vi "New Template - Test Plan Template (SubVI).vi"(8 "error in":errorcluster, 9 "Load path":path, 10 "File Name:":string, 11 "Test Type":T1 items=["Please Select", "Triaxial Shear", "Triaxial UU", "Shearbox", "Permeability", "Consolidation (Stepped Loading)/Swelling", "Saturation (Incremental)", "User Defined", "UCT", "Isotropic Consolidation", "Swelling Pressure"]) -> (0 "error out":errorcluster)   [LabVIEW 2019]
uses:
  Controls/Test Plan - Start Conditions Tab.ctl
  Controls/Test Plan - Stop Conditions Tab.ctl
  Controls/Test Plan - Log Conditions Tab.ctl
  Controls/Station - Test Type.ctl
  Controls/Test Plan Template - State.ctl
panel:
  in  "Save":bool
  in  "Tab con":T2(tab)
  in  "Start Enable":bool
  out "Start Tab":T3=enum."User Defined"
  in  "Cons Start VS":dbl caption="N"
  in  "Cons Start Delay":timestamp format="%<%H:%M:%S>T"
  in  "Cons Start .Delay":bool
  in  "Sat Start BP":bool
  in  "Sat BP":dbl caption="kPa"
  in  "Sat CP":dbl caption="kPa"
  in  "Iso BP":dbl caption="kPa"
  in  "Start Load":string[][](table) caption="Use the following table for consolidation pressure:"
  in  "Start load":dbl format="%#_13g"
  in  "Start Delay":u32
  in  "Sub Start":enum32{"1", "2"}(radio)
  in  "TS Drain":enum32{"1", "2"}(radio)
  in  "TS Engage":bool
  in  "TS Load Change":dbl caption="N"
  in  "TS Engage Speed":dbl caption="mm/min"
  in  "TS Shear Speed":dbl caption="mm/min"
  in  "TUU Start Delay":timestamp format="%<%H:%M:%S>T"
  in  "TUU Start .Delay":bool
  in  "TUU Confining Pressure":dbl caption="kPa"
  in  "TUU Engage":bool
  in  "TUU Load Change":dbl caption="N"
  in  "TUU Engage Speed":dbl caption="mm/min"
  in  "TUU Shear Speed":dbl caption="mm/min"
  in  "UCT Engage":bool
  in  "UCT Load Change":dbl caption="N"
  in  "UCT Engage Speed":dbl caption="mm/min"
  in  "UCT Shear Speed":dbl caption="mm/min"
  in  "SB Start Delay":timestamp format="%<%H:%M:%S>T"
  in  "SB Start .Delay":bool
  in  "SB Vertical Load":dbl caption="N"
  in  "SB Engage":bool
  in  "SB Load Change":dbl caption="N"
  in  "SB Engage Speed":dbl caption="mm/min"
  in  "SB Shear Speed":dbl caption="mm/min"
  in  "Perm DP":dbl caption="kPa"
  out "Log Tab":T4=enum."User Defined"
  in  "Cons Log Select":enum32{"1", "2"}(radio)
  out "ConsTable":enum32{"None", "Time", "Disp"}(tab)
  in  "Cons LogTime":string[][](table)
  in  "Cons LogDisp":string[][](table)
  in  "Cons Log Delay":timestamp format="%<%H:%M:%S>T"
  in  "Sat Log Delay":timestamp format="%<%H:%M:%S>T"
  out "SatTable":enum32{"None", "Time", "Disp"}(tab)
  in  "Sat LogTime":string[][](table)
  in  "Sat LogDisp":string[][](table)
  in  "Sat Log Select":enum32{"1", "2"}(radio)
  in  "Iso Log Select":enum32{"1", "2"}(radio)
  out "IsoTable":enum32{"None", "Time", "Disp"}(tab)
  in  "Iso LogTime":string[][](table)
  in  "Iso LogDisp":string[][](table)
  in  "Iso Log Delay":timestamp format="%<%H:%M:%S>T"
  in  "LOG delay":u32
  out "LOG Table":enum32{"None", "Time", "Disp"}(tab)
  in  "LOG Time":string[][](table)
  in  "LOG Disp":string[][](table)
  in  "Sub Log":enum32{"1", "2", "3"}(radio)
  in  "Log VL":u16(ring) caption="Vertical Load(Kpa)" items=["Please select"]
  in  "SET":bool
  in  "TS LogAxial":sgl
  in  "TS Log Delay":timestamp format="%<%H:%M:%S>T"
  out "TSTable":enum32{"None", "Time", "Disp"}(tab)
  in  "TS LogTime":string[][](table)
  in  "TS LogDisp":string[][](table)
  in  "TS Log Select":enum32{"1", "3", "2"}(radio)
  in  "TUU LogAxial":sgl
  in  "TUU Log Delay":timestamp format="%<%H:%M:%S>T"
  out "TUUTable":enum32{"None", "Time", "Disp"}(tab)
  in  "TUU LogTime":string[][](table)
  in  "TUU LogDisp":string[][](table)
  in  "TUU Log Select":enum32{"1", "3", "2"}(radio)
  in  "UCT LogAxial":sgl
  in  "UCT Log Delay":timestamp format="%<%H:%M:%S>T"
  out "UCTTable":enum32{"None", "Time", "Disp"}(tab)
  in  "UCT LogTime":string[][](table)
  in  "UCT LogDisp":string[][](table)
  in  "UCT Log Select":enum32{"1", "3", "2"}(radio)
  in  "SB Log Delay":timestamp format="%<%H:%M:%S>T"
  out "SBTable":enum32{"None", "Time", "Disp"}(tab)
  in  "SB LogTime":string[][](table)
  in  "SB LogDisp":string[][](table)
  in  "SB Log Select":enum32{"1", "2"}(radio)
  in  "Perm Log Delay":timestamp format="%<%H:%M:%S>T"
  in  "Perm Log Select":enum32{"1"}(radio)
  in  "SP Log Delay":timestamp format="%<%H:%M:%S>T"
  in  "SP Log Select":enum32{"1"}(radio)
  in  "Stop Enable":bool
  out "Stop Tab":T5=enum."User Defined"
  in  "Cons Stop Swell":bool caption="When swelling is detected by the amount given"
  in  "Cons Stop Time":timestamp format="%<%H:%M:%S>T"
  in  "Cons Stop Time2":string="00:00:00"
  in  "Cons Stop Select":enum32{"1", "2"}(radio)
  in  "Cons Stop Disp":dbl caption="mm"
  in  "Cons Stop Disp 2":dbl caption="mm"
  in  "Sat Stop Time3":string="00:00:00"
  in  "Sat Stop VC":dbl caption="cm3"
  in  "Sat Stop PP":dbl caption="kPa"
  in  "Sat Stop Select":enum32{"1", "2", "3"}(radio)
  in  "Sat Stop Time2":timestamp format="%<%H:%M:%S>T"
  in  "Sat Stop Time":timestamp format="%<%H:%M:%S>T"
  in  "Sat Stop B":dbl caption="%" format="%.2f"
  in  "Sat Stop .B":bool
  in  "Iso Stop Time":string="00:00:00"
  in  "Iso Stop Select":enum32{"1", "2"}(radio)
  in  "Iso Stop Time2":timestamp format="%<%H:%M:%S>T"
  in  "Iso Stop PP":dbl caption="%"
  in  "Iso Stop VC":dbl caption="cm3"
  in  "Iso Stop .PP":bool
  in  "Return":bool
  in  "Stop Time":timestamp=timestamp(57600 s since 1904-01-01) format="%<%H:%M:%S>T"
  in  "Stop Duration":u32
  in  "stop load":dbl format="%#_13g"
  in  "Sub Stop":enum32{"1", "2"}(radio)
  in  "TS Reset Value":dbl caption="%"
  in  "TS Axial Value":dbl caption="%"
  in  "TS MaxDev":bool
  in  "TS MaxDev Value":dbl caption="%"
  in  "TS Reset":bool
  in  "TS Return":bool
  in  "TUU Reset Value":dbl caption="%"
  in  "TUU Axial Value":dbl caption="%"
  in  "TUU MaxDev":bool
  in  "TUU MaxDev Value":dbl caption="%"
  in  "TUU Reset":bool
  in  "TUU Return":bool
  in  "UCT Reset Value":dbl caption="%"
  in  "UCT Axial Value":dbl caption="%"
  in  "UCT MaxDev":bool
  in  "UCT MaxDev Value":dbl caption="%"
  in  "UCT Reset":bool
  in  "UCT Return":bool
  in  "SB Reset Value":dbl caption="%"
  in  "SB Shear Value":dbl caption="%"
  in  "SB MaxShear":bool
  in  "SB MaxShear Value":dbl caption="%"
  in  "SB Reset":bool
  in  "SB Return":bool
  in  "Perm Ratio More":dbl caption="%"
  in  "Perm Ratio Time":string="00:00:00"
  in  "Perm Stop Time":string="00:00:00"
  in  "Perm Reset Value":dbl caption="%"
  in  "Perm Ratio Less":dbl caption="%"
  in  "Perm MaxTime":bool
  in  "Perm Reset":bool
  in  "Perm Ratio":bool
  in  "SP Stop Time":string="00:00:00"
  in  "SP Stop Max Time":string="00:00:00"
  in  "SP Stop Stress":dbl caption="%"
  in  "SP Stop .MaxTime":bool
  in  "SP Stop .Time":bool
  # "Vertical Load will be :"
  # "Wait until the following delay expires"
  # "Cell Pressure will be :"
  # "Back Pressure will be :"
  # "Hold Back Pressure at :"
  # "Shear speed will be:"
  # "Engage Speed :"
  # "Until the load changes by"
  # "Wait until the following delay expires"
  # "Confining Pressure will be:"
  # "Shear speed will be:"
  # "Engage Speed :"
  # "Until the load changes by"
  # "Shear speed will be:"
  # "Engage Speed :"
  # "Until the load changes by"
  # "Wait until the following delay expires"
  # "Vertical Load will be:"
  # "Shear speed will be:"
  # "Engage Speed :"
  # "Until the load changes by"
  # "Drain Pressure will be:"
  # "Data will be logged as soon as the test is started"
  # "B value is above this level"
  # "When the Pore Pressure Dissipation exceeds the\npercentage entered here"
  # "When the Axial Strain extends beyond the\npercentage entered here"
  # "When the Maximum Deviator Stress falls by the\npercentage entered here"
  # "Return the load frame to home position"
  # "Reset Cell And Back Pressure Control to amount\nentered here"
  # "When the Axial Strain extends beyond the\npercentage entered here"
  # "When the Maximum Deviator Stress falls by the\npercentage entered here"
  # "Return the load frame to home position"
  # "Reset Cell Pressure Control to amount\nentered here"
  # "When the Axial Strain extends beyond the\npercentage entered here"
  # "When the Maximum Deviator Stress falls by the\npercentage entered here"
  # "Return the load frame to home position"
  # "When the Shear Strain extends beyond the\npercentage entered here"
  # "When the Maximum Shear Stress falls by the\npercentage entered here"
  # "Return the Horizontal piston to home position"
  # "Reset Vertical Load to amount\nentered here"
  # "<= Ratio <="
  # "When the top and bottom volume change is steady\n(constant flow) over the period of time entered here"
  # "When the maximum time entered here is exceeded"
  # "Reset Drain Pressure, Back Pressure and\nCell Pressure to amount entered here"
  # "Stop when the Specimen Stress Changes by less  than \nthis amount during the following interval : (kPa/time)"
  # "When the maximum time entered here is exceeded"
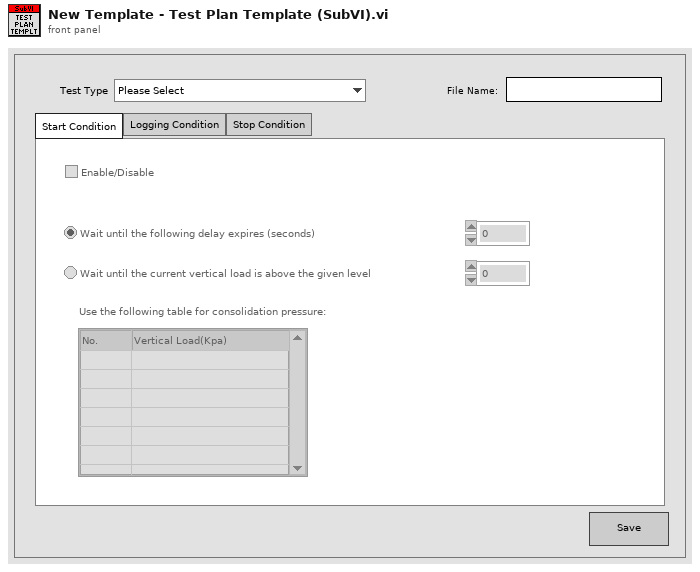
[diagram p1: front panel]
types:
  T1 = typedef "Station - Test Type.ctl" = u16
  T2 = enum32{"Start Condition", "Logging Condition", "Stop Condition"}
  T3 = typedef "Test Plan - Start Conditions Tab.ctl" = enum32{"Consolidation", "Saturation", "Iso Consolidation", "User Defined", "Others", "TS", "TUU", "UCT", "Shearbox", "Permiability", "SP"}
  T4 = typedef "Test Plan - Log Conditions Tab.ctl" = enum32{"Consolidation", "Saturation", "Iso Consolidation", "User Defined", "Others", "TS", "TUU", "UCT", "Shearbox", "Permiability", "SP"}
  T5 = typedef "Test Plan - Stop Conditions Tab.ctl" = enum32{"Consolidation", "Saturation", "Iso Consolidation", "User Defined", "Others", "TS", "TUU", "UCT", "Shearbox", "Permiability", "SP"}
  T6 = typedef "Test Plan Template - State.ctl" = enum16{"Init", "Idle", "Load VL", "Load Start", "Load Log", "Load Stop", "Load Device", "Save", "Close"}
  T7 = enum8{"Enabled", "Disabled", "Disabled and Grayed Out"}
  T8 = cluster{"TestPlan Section":string, "Key Value":string[]}[]
  T9 = cluster{"TestPlan Section":string, "Key Value":string[]}
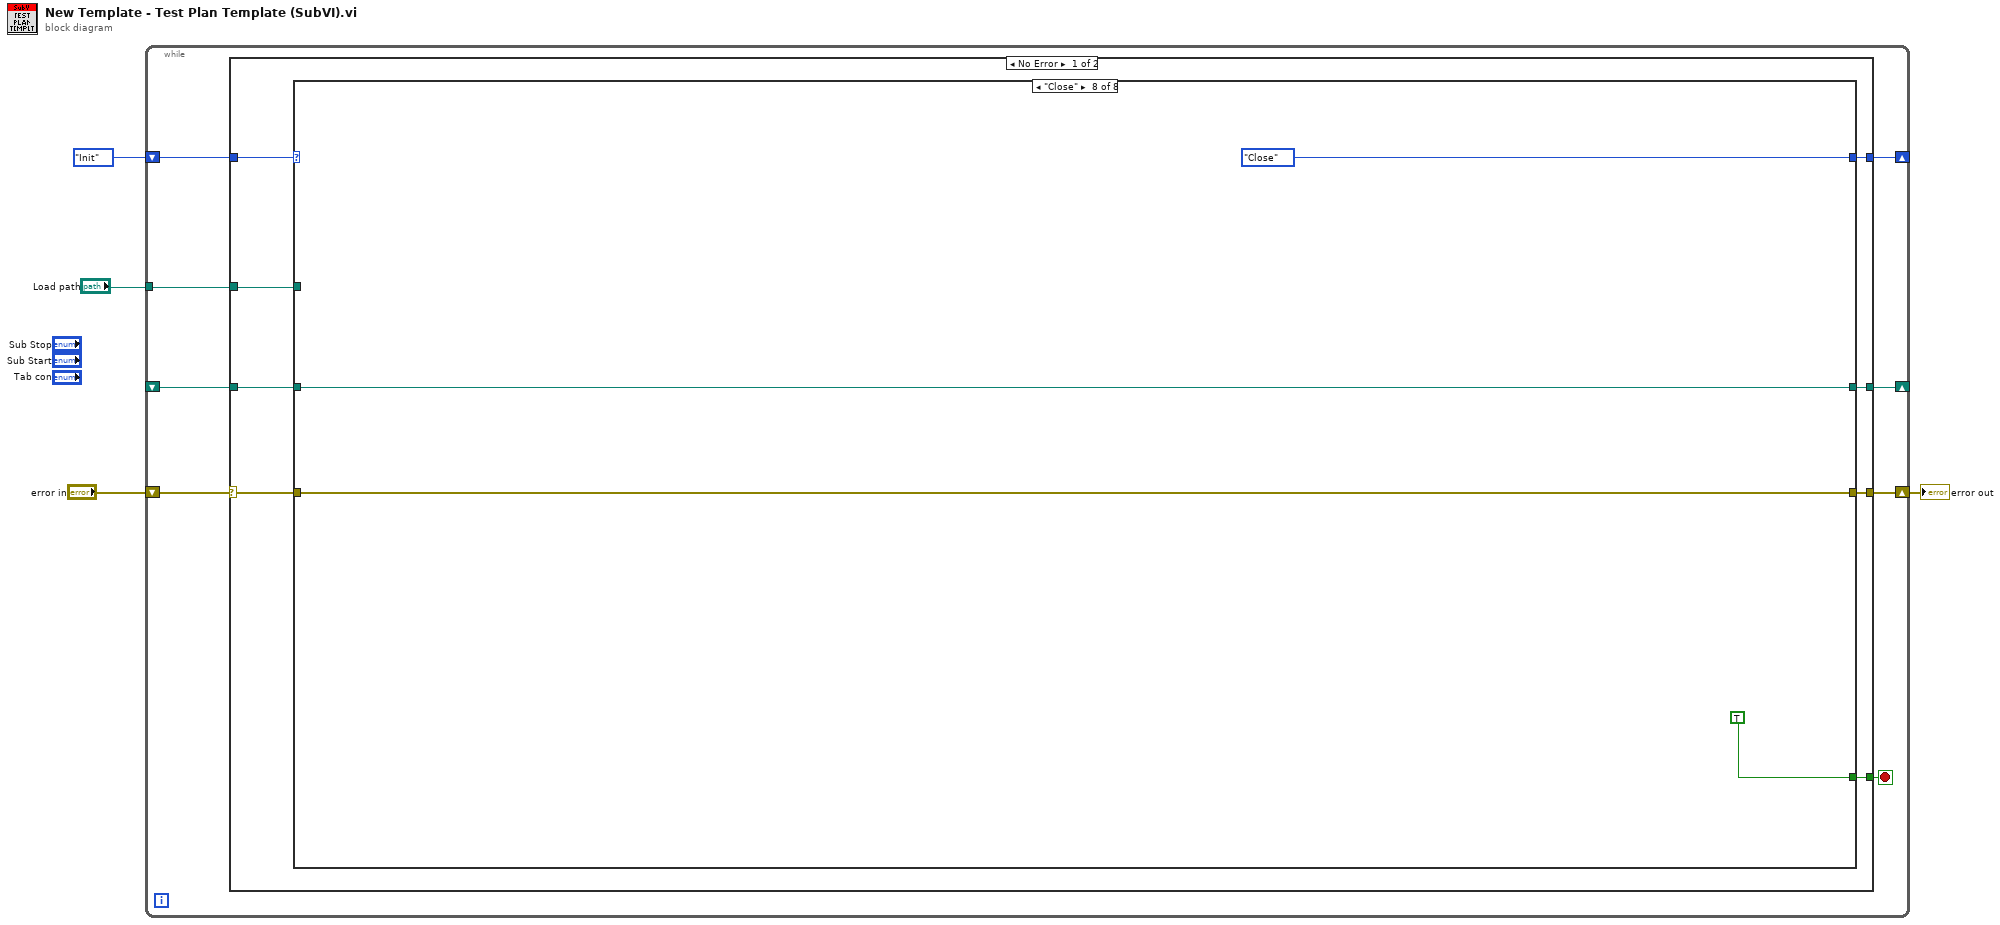
[diagram p0: block diagram]
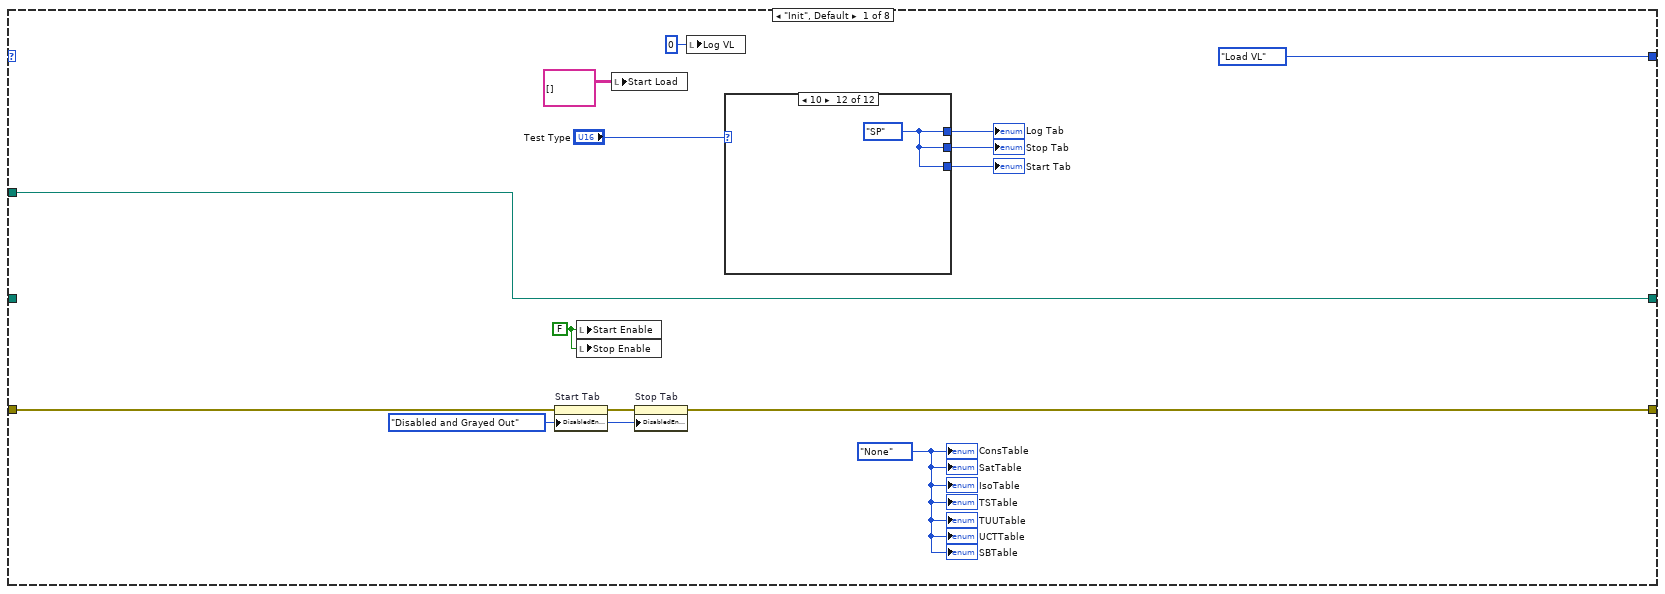
[diagram p2: hidden frame]
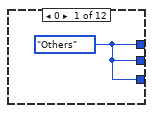
[diagram p3: hidden frame]
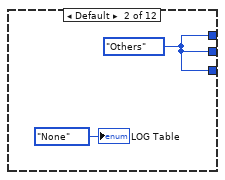
[diagram p4: hidden frame]
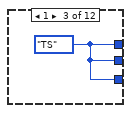
[diagram p5: hidden frame]
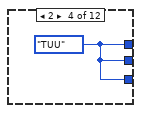
[diagram p6: hidden frame]
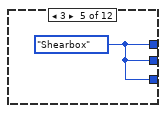
[diagram p7: hidden frame]
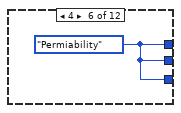
[diagram p8: hidden frame]
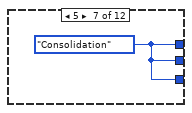
[diagram p9: hidden frame]
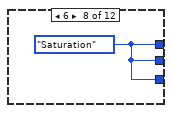
[diagram p10: hidden frame]
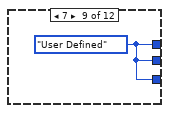
[diagram p11: hidden frame]
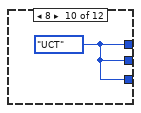
[diagram p12: hidden frame]
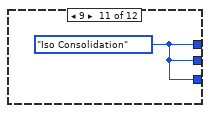
[diagram p13: hidden frame]
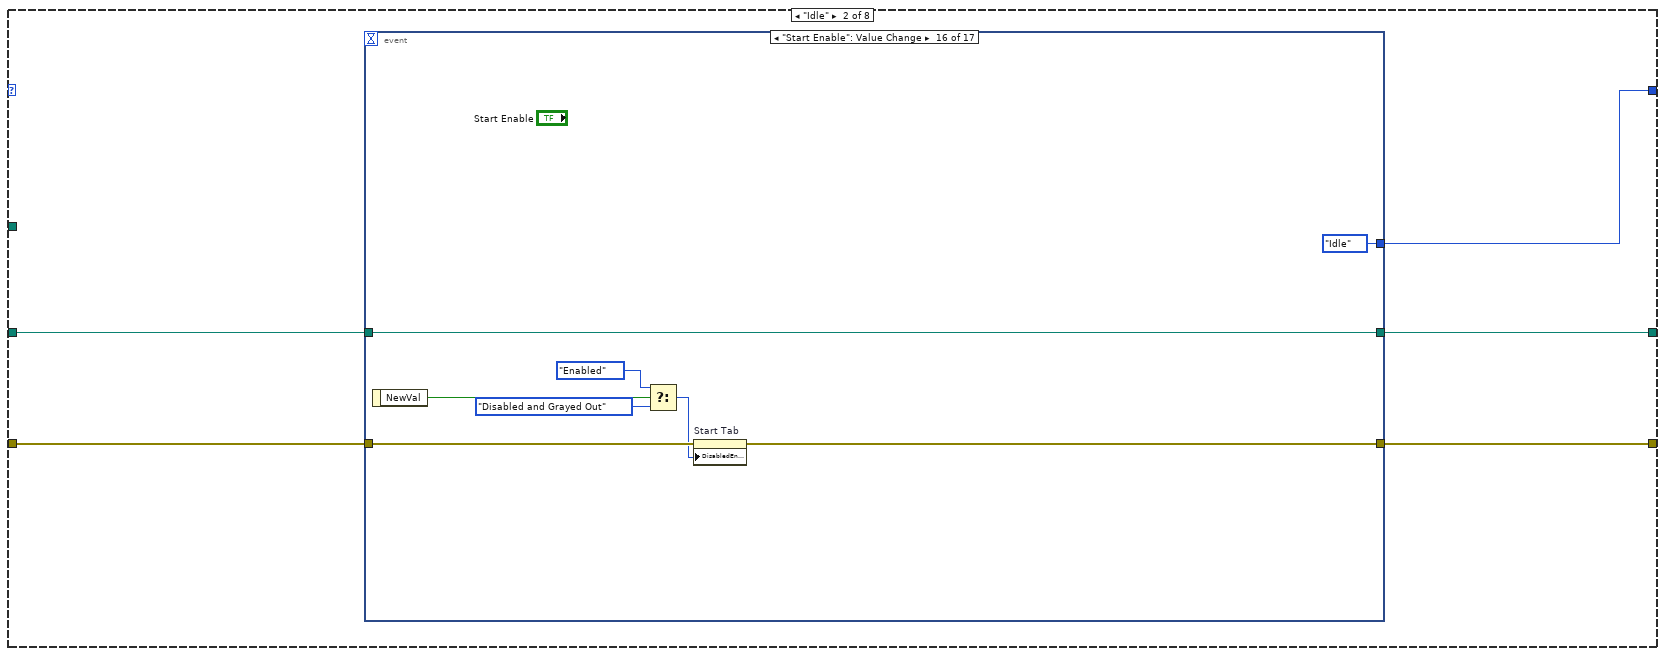
[diagram p14: hidden frame]
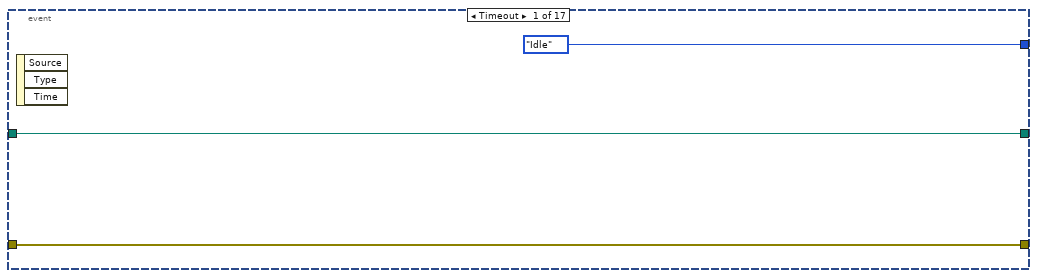
[diagram p15: hidden frame]
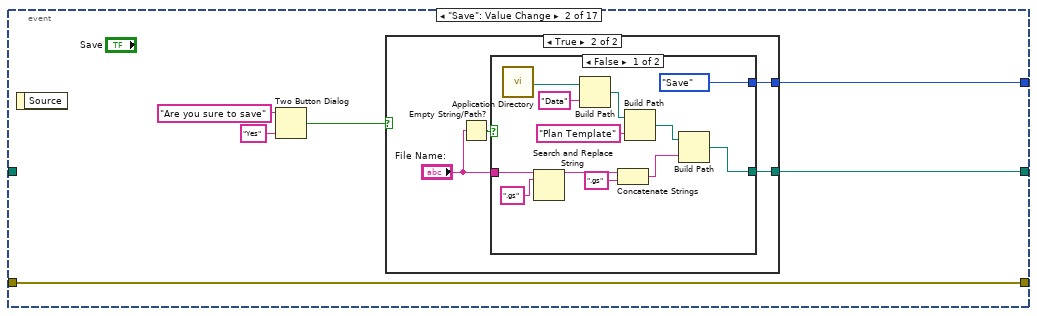
[diagram p16: hidden frame]
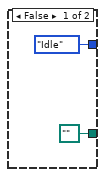
[diagram p17: hidden frame]
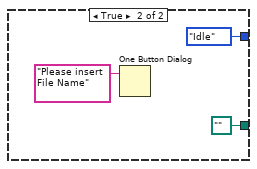
[diagram p18: hidden frame]
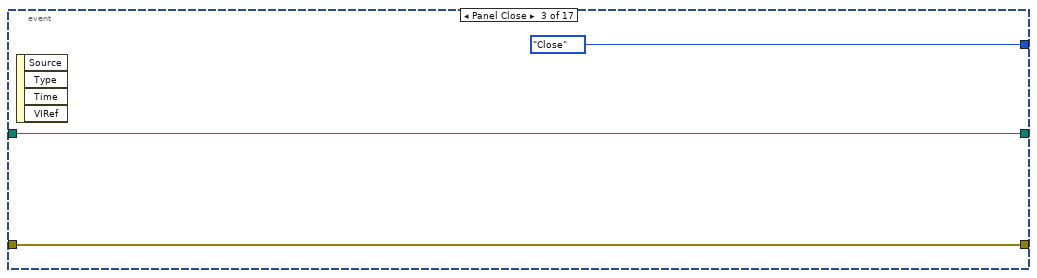
[diagram p19: hidden frame]
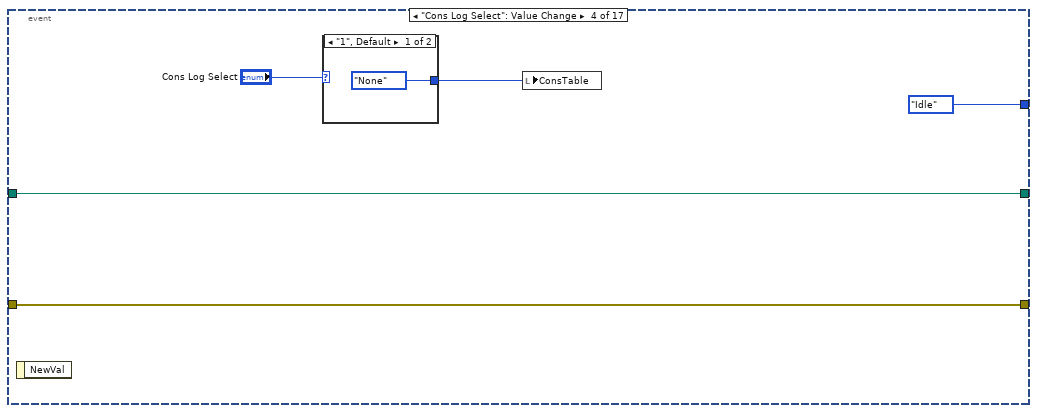
[diagram p20: hidden frame]
diagram:
  n1 = while {
    shift-right: [w12] -> w4
    shift-left: "error in" -> [w11]
    shift-right: [w9] -> _
    shift-left: Test_Plan_Template_-_State."Init" -> [w10]
    shift-right: [w8] -> _
    shift-left: _ -> [w7]
    tunnel: "Load path" -> [w5]
    stop <- w6 stop-if-true
    n2 = case shown="No Error" w11 {
      selector: w11 -> [w19 w1656]
      tunnel: [w20 w1655] -> w12
      tunnel: w10 -> [w18 _]
      tunnel: [w17 Test_Plan_Template_-_State."Idle" ("Enum")] -> w9
      tunnel: [w16 w1652] -> w8
      tunnel: w7 -> [w15 w1652]
      tunnel: [w14 _] -> w6
      tunnel: w5 -> [w13 _]
      frame No Error {
        n3 = case shown="\"Close\"" w18 {
          tunnel: [w24 w52 w264 w291 w471 w789 w1121 w1651] -> w20
          tunnel: w19 -> [w23 w51 w269 w296 w476 w794 w1126 w1651]
          tunnel: [Test_Plan_Template_-_State."Load VL" w50 Test_Plan_Template_-_State."Load Start" ("Enum") Test_Plan_Template_-_State."Load Log" ("Enum") Test_Plan_Template_-_State."Load Stop" ("Enum") Test_Plan_Template_-_State."Idle" ("Enum") w1120 Test_Plan_Template_-_State."Close" ("Enum")] -> w17
          tunnel: [w30 w49 w266 w293 w473 w791 w1123 w1650] -> w16
          tunnel: w15 -> [_ w48 w265 w292 w472 w790 w1123 w1650]
          tunnel: [_ _ _ _ _ _ _ TRUE] -> w14
          tunnel: w13 -> [w30 _ w268 w295 w475 w793 _ _]
          frame "Init", Default {
            w22 = T7."Disabled and Grayed Out" ("Disabled")
            w26 = FALSE ("Start Enable")
            w21 = enum32{"None", "Time", "Disp"}."None" ("CustomTable")
            n4 = property on="Start Tab" class="TabCtl (strict)"(error in=w23, "DisabledEnum"=w22) -> (error out=w25:errorcluster)  [unwired: 1 in, 1 out]
            n5 = local write "Start Enable"(w26) -> ()
            n6 = local write "Stop Enable"(w26) -> ()
            n7 = local write "Start Load"(string[][] [] ("Start 1DLoad")) -> ()
            n8 = property on="Stop Tab" class="TabCtl (strict)"(error in=w25, "DisabledEnum"=w22) -> (error out=w24:errorcluster)  [unwired: 1 in, 1 out]
            n9 = local write "Log VL"(0) -> ()
            n10 = case shown="10" "Test Type" {
              tunnel: [w35 w36 w38 w39 w40 w41 w42 w43 w44 w45 w46 w47] -> w29
              tunnel: [w35 w36 w38 w39 w40 w41 w42 w43 w44 w45 w46 w47] -> w28
              tunnel: [w35 w36 w38 w39 w40 w41 w42 w43 w44 w45 w46 w47] -> w27
              frame 0 {
                w35 = Test_Plan_-_Log_Conditions_Tab."Others" ("Log Tab")
              }
              frame Default {
                w36 = Test_Plan_-_Log_Conditions_Tab."Others" ("Log Tab")
                "LOG Table" <- enum32{"None", "Time", "Disp"}."None" ("1DTable")
              }
              frame 1 {
                w38 = Test_Plan_-_Log_Conditions_Tab."TS" ("Log Tab")
              }
              frame 2 {
                w39 = Test_Plan_-_Log_Conditions_Tab."TUU" ("Log Tab")
              }
              frame 3 {
                w40 = Test_Plan_-_Log_Conditions_Tab."Shearbox" ("Log Tab")
              }
              frame 4 {
                w41 = Test_Plan_-_Log_Conditions_Tab."Permiability" ("Log Tab")
              }
              frame 5 {
                w42 = Test_Plan_-_Log_Conditions_Tab."Consolidation" ("Log Tab")
              }
              frame 6 {
                w43 = Test_Plan_-_Log_Conditions_Tab."Saturation" ("Log Tab")
              }
              frame 7 {
                w44 = Test_Plan_-_Log_Conditions_Tab."User Defined" ("Log Tab")
              }
              frame 8 {
                w45 = Test_Plan_-_Log_Conditions_Tab."UCT" ("Log Tab")
              }
              frame 9 {
                w46 = Test_Plan_-_Log_Conditions_Tab."Iso Consolidation" ("Log Tab")
              }
              frame 10 {
                w47 = Test_Plan_-_Log_Conditions_Tab."SP" ("Log Tab")
              }
            }
            "Log Tab" <- w29
            "Stop Tab" <- w28
            "Start Tab" <- w27
            "ConsTable" <- w21
            "SatTable" <- w21
            "IsoTable" <- w21
            "TSTable" <- w21
            "TUUTable" <- w21
            "UCTTable" <- w21
            "SBTable" <- w21
          }
          frame "Idle" {
            n11 = event shown="[15] \"Start Enable\": Value Change" {
              selector: _ -> [_ _ _ _ _ _ _ _ _ _ _ _ _ _ _ _ _]
              dyn-events: _ -> [_ _ _ _ _ _ _ _ _ _ _ _ _ _ _ _ _]
              timeout: _ -> [_ _ _ _ _ _ _ _ _ _ _ _ _ _ _ _ _]
              tunnel: [w55 w60 w85 w88 w95 w102 w109 w116 w123 w128 w131 w136 w141 w215 w246 w253 w259] -> w52
              tunnel: w51 -> [w55 w60 w85 w88 w95 w102 w109 w116 w123 w128 w131 w136 w152 w237 w246 w252 w258]
              tunnel: [Test_Plan_Template_-_State."Idle" w61 Test_Plan_Template_-_State."Close" ("Enum") Test_Plan_Template_-_State."Idle" ("Enum") Test_Plan_Template_-_State."Idle" ("Enum") Test_Plan_Template_-_State."Idle" ("Enum") Test_Plan_Template_-_State."Idle" ("Enum") Test_Plan_Template_-_State."Idle" ("Enum") Test_Plan_Template_-_State."Idle" ("Enum") Test_Plan_Template_-_State."Idle" ("Enum") Test_Plan_Template_-_State."Idle" ("Enum") Test_Plan_Template_-_State."Idle" ("Enum") Test_Plan_Template_-_State."Idle" ("Enum") Test_Plan_Template_-_State."Idle" ("Enum") Test_Plan_Template_-_State."Idle" ("Enum") Test_Plan_Template_-_State."Idle" ("Enum") Test_Plan_Template_-_State."Idle" ("Enum")] -> w50
              tunnel: [w53 w59 w84 w90 w97 w104 w111 w118 w125 w130 w133 w138 w151 w216 w247 w255 w263] -> w49
              tunnel: w48 -> [w53 _ w84 w90 w97 w104 w111 w118 w125 w130 w133 w138 w151 w216 w247 w255 w263]
              event Timeout {
                n12 = event-data() -> ()  [unwired: 1 in, 3 out]
              }
              event "Save": Value Change {
                n13 = event-data() -> ()  [unwired: 1 in, 1 out]
                n14 = Two Button Dialog(message="Are you sure to save", 2:"Yes" ("T button name (\"OK\")")) -> (T button?=w58:bool)  [unwired: 1 in]
                n15 = case shown="True" w58 {
                  tunnel: [Test_Plan_Template_-_State."Idle" ("Enum") w67] -> w61
                  tunnel: [path "" ("appended path") w64] -> w59
                  frame False {
                  }
                  frame True {
                    n16 = Empty String/Path?(string/path="File Name:") -> (empty?=w65:bool)
                    n17 = case shown="False" w65 {
                      tunnel: [Test_Plan_Template_-_State."Save" ("Enum") Test_Plan_Template_-_State."Idle" ("Enum")] -> w67
                      tunnel: "File Name:" -> [w72 _]
                      tunnel: [w74 path "" ("appended path")] -> w64
                      frame False {
                        n18 = call <vilib>:"Application Directory.vi"() -> ("Application Directory"=w70:path)
                        n19 = Search and Replace String(input string=w72, search string=".gs") -> (result string=w73:string)  [unwired: 6 in, 3 out]
                        n20 = Build Path(base path=w70, name or relative path="Data") -> (appended path=w68:path)
                        n21 = Concatenate Strings(w73, ".gs" ("string")) -> (w78:string)
                        n22 = Build Path(base path=w68, name or relative path="Plan Template") -> (appended path=w77:path)
                        n23 = Build Path(base path=w77, name or relative path=w78) -> (appended path=w74:path)
                      }
                      frame True {
                        n24 = One Button Dialog(message="Please insert File Name") -> ()  [unwired: 1 in, 1 out]
                      }
                    }
                  }
                }
              }
              event Panel Close {
                n25 = event-data() -> ()  [unwired: 1 in, 4 out]
              }
              event "Cons Log Select": Value Change {
                n26 = event-data() -> ()  [unwired: 1 in, 1 out]
                n27 = case shown="\"1\", Default" "Cons Log Select" {
                  tunnel: [enum32{"None", "Time", "Disp"}."None" ("ConsTable") enum32{"None", "Time", "Disp"}."Time" ("ConsTable")] -> w86
                  frame "1", Default {
                  }
                  frame "2" {
                  }
                }
                n28 = local write "ConsTable"(w86) -> ()
              }
              event "Sat Log Select": Value Change {
                n29 = event-data() -> ()  [unwired: 1 in, 1 out]
                n30 = case shown="\"2\"" "Sat Log Select" {
                  tunnel: [enum32{"None", "Time", "Disp"}."None" ("ConsTable") enum32{"None", "Time", "Disp"}."Time" ("ConsTable")] -> w93
                  frame "1", Default {
                  }
                  frame "2" {
                  }
                }
                n31 = local write "SatTable"(w93) -> ()
              }
              event "Iso Log Select": Value Change {
                n32 = event-data() -> ()  [unwired: 1 in, 1 out]
                n33 = case shown="\"2\"" "Iso Log Select" {
                  tunnel: [enum32{"None", "Time", "Disp"}."None" ("ConsTable") enum32{"None", "Time", "Disp"}."Time" ("ConsTable")] -> w100
                  frame "1", Default {
                  }
                  frame "2" {
                  }
                }
                n34 = local write "IsoTable"(w100) -> ()
              }
              event "TS Log Select": Value Change {
                n35 = event-data() -> ()  [unwired: 1 in, 6 out]
                n36 = case shown="\"3\"" "TS Log Select" {
                  tunnel: [enum32{"None", "Time", "Disp"}."None" ("ConsTable") enum32{"None", "Time", "Disp"}."Disp" ("ConsTable")] -> w107
                  frame "1", Default {
                  }
                  frame "3" {
                  }
                }
                n37 = local write "TSTable"(w107) -> ()
              }
              event "TUU Log Select": Value Change {
                n38 = event-data() -> ()  [unwired: 1 in, 6 out]
                n39 = case shown="\"3\"" "TUU Log Select" {
                  tunnel: [enum32{"None", "Time", "Disp"}."None" ("ConsTable") enum32{"None", "Time", "Disp"}."Disp" ("ConsTable")] -> w114
                  frame "1", Default {
                  }
                  frame "3" {
                  }
                }
                n40 = local write "TUUTable"(w114) -> ()
              }
              event "SB Log Select": Value Change {
                n41 = event-data() -> ()  [unwired: 1 in, 6 out]
                n42 = case shown="\"2\"" "SB Log Select" {
                  tunnel: [enum32{"None", "Time", "Disp"}."None" ("ConsTable") enum32{"None", "Time", "Disp"}."Disp" ("ConsTable")] -> w122
                  frame "1", Default {
                  }
                  frame "2" {
                  }
                }
                n43 = local write "SBTable"(w122) -> ()
              }
              event "Perm Log Select": Value Change {
                n44 = event-data() -> ()  [unwired: 1 in, 6 out]
              }
              event "SP Log Select": Value Change {
                n45 = event-data() -> ()  [unwired: 1 in, 6 out]
              }
              event "UCT Log Select": Value Change {
                n46 = event-data() -> ()  [unwired: 1 in, 6 out]
                n47 = case shown="\"3\"" "UCT Log Select" {
                  tunnel: [enum32{"None", "Time", "Disp"}."None" ("ConsTable") enum32{"None", "Time", "Disp"}."Disp" ("ConsTable")] -> w134
                  frame "1", Default {
                  }
                  frame "3" {
                  }
                }
                n48 = local write "UCTTable"(w134) -> ()
              }
              event "Log VL": Value Change {
                n49 = event-data() -> ()  [unwired: 1 in, 1 out]
                n50 = call "TestPlan - Config File.vi"("Action"=enum16{"Write", "Read", "Read All", "Remove"}."Read", "file path"=w151, "error in (no error)"=w152, "TestPlan Section"="Log VL" ("TestPlan Name")) -> ("error out"=w149:errorcluster, "key names"=w146:string[], "Value Out"=w145:T8)  [unwired: 5 in]
                n51 = property on="Log VL" class="Ring (strict)"(error in=w149) -> (error out=w142:errorcluster, "RingText.Text"=w147:string)  [unwired: 1 in, 1 out]
                n52 = Index Array(array=w145, index=0) -> (element=w143:T9)
                n53 = for {
                  N: 4 -> [_]
                  tunnel: w147 -> [w167]
                  tunnel: w146 -> [w165]
                  tunnel: w143 -> [w163]
                  shift-right: [w157] -> w141
                  shift-left: w142 -> [w160]
                  i -> [w159]
                  n54 = Unbundle By Name(w163) -> ("Key Value"=w162:string[])
                  n55 = Format Into String(format string="-%d", initial string=w167, error in=w160, w159) -> (resulting string=w164:string, error out=w158:errorcluster)
                  n56 = Search 1D Array(1D array=w165, element=w164) -> (index of element=w161:i32)  [unwired: 1 in]
                  n57 = Index Array(array=w162, index=w161) -> (element=w156:string)
                  n58 = case shown="3" w159 {
                    tunnel: w158 -> [w171 w174 w177 w193]
                    tunnel: [w170 w174 w178 w194] -> w157
                    tunnel: w156 -> [w169 w173 w182 w198]
                    tunnel: string[] [] ("array type (2D Dbl)") -> [_ _ w180 w196]
                    frame 0, Default {
                      n59 = Decimal String To Number(string=w169) -> (number=w168:i32)  [unwired: 2 in, 1 out]
                      n60 = local write "LOG Table"(w168) -> ()
                      n61 = property on="Sub Log" class="RadioBtnsControl (strict)"(error in=w171, "Val(Sgnl)"=w168) -> (error out=w170:errorcluster)  [unwired: 1 in, 1 out]
                    }
                    frame 1 {
                      n62 = Decimal String To Number(string=w173) -> (number=w172:i32)  [unwired: 2 in, 1 out]
                      n63 = local write "LOG delay"(w172) -> ()
                    }
                    frame 2 {
                      n64 = Spreadsheet String To Array(delimiter (Tab)=",", format string="", spreadsheet string=w182, array type (2D Dbl)=w180) -> (array=w179:string[])
                      n65 = for {
                        tunnel: w179 -> [w185] mode=indexing
                        shift-right: [w188] -> w178
                        shift-left: w177 -> [w189]
                        tunnel: [w183] -> w176 mode=indexing
                        i -> [w187]
                        n66 = Increment(x=w187) -> (x+1=w186:i32)
                        n67 = Format Into String(format string="%d", error in=w189, w186) -> (resulting string=w184:string, error out=w188:errorcluster)  [unwired: 1 in]
                        n68 = Build Array(w184, w185) -> (w183:string[])
                      }
                      n69 = local write "LOG Time"(w176) -> ()
                    }
                    frame 3 {
                      n70 = Spreadsheet String To Array(delimiter (Tab)=",", format string="", spreadsheet string=w198, array type (2D Dbl)=w196) -> (array=w195:string[])
                      n71 = for {
                        tunnel: w195 -> [w201] mode=indexing
                        shift-right: [w204] -> w194
                        shift-left: w193 -> [w205]
                        tunnel: [w199] -> w192 mode=indexing
                        i -> [w203]
                        n72 = Increment(x=w203) -> (x+1=w202:i32)
                        n73 = Format Into String(format string="%d", error in=w205, w202) -> (resulting string=w200:string, error out=w204:errorcluster)  [unwired: 1 in]
                        n74 = Build Array(w200, w201) -> (w199:string[])
                      }
                      n75 = local write "LOG Disp"(w192) -> ()
                    }
                  }
                }
              }
              event "SET": Value Change {
                n76 = event-data() -> ()  [unwired: 1 in, 1 out]
                n77 = property on="Log VL" class="Ring (strict)"(error in=w237) -> (error out=w217:errorcluster, "RingText.Text"=w218:string)  [unwired: 1 in, 1 out]
                n78 = local read "Sub Log"() -> (w232:enum32{"1", "2", "3"})
                n79 = for {
                  N: 4 -> [_]
                  tunnel: w218 -> [w241]
                  tunnel: [w239] -> w235 mode=indexing
                  i -> [w242]
                  n80 = Format Into String(format string="-%d", initial string=w241, w242) -> (resulting string=w239:string)  [unwired: 1 in, 1 out]
                }
                n81 = To Unsigned Word Integer(number=w232) -> (unsigned 16bit integer=w233:u16)
                n82 = Number To Decimal String(number=w233) -> (decimal integer string=w234:string)  [unwired: 1 in]
                n83 = Number To Decimal String(number="LOG delay") -> (decimal integer string=w229:string)  [unwired: 1 in]
                n84 = Index Array(array="LOG Time", index (col)=1 ("disabled index (col)")) -> (element=w210:string[])  [unwired: 1 in]
                n85 = Index Array(array="LOG Disp", index (col)=1 ("disabled index (col)")) -> (element=w208:string[])  [unwired: 1 in]
                n86 = call "Test Plan - Remove Empty Element (SubVI).vi"("Data"=w210) -> ("Result"=w209:string[])  [unwired: 10 in]
                n87 = call "Test Plan - Remove Empty Element (SubVI).vi"("Data"=w208) -> ("Result"=w207:string[])  [unwired: 10 in]
                n88 = Array To Spreadsheet String(delimiter (Tab)=",", array=w209, 3:"" ("format string")) -> (spreadsheet string=w230:string)
                n89 = Array To Spreadsheet String(delimiter (Tab)=",", array=w207, 3:"" ("format string")) -> (spreadsheet string=w231:string)
                n90 = call <vilib>:"Trim Whitespace.vi"("string"=w230) -> ("trimmed string"=w212:string)  [unwired: 1 in]
                n91 = call <vilib>:"Trim Whitespace.vi"("string"=w231) -> ("trimmed string"=w211:string)  [unwired: 1 in]
                n92 = Build Array(w234, w229, w212, w211) -> (w236:string[])
                n93 = call "TestPlan - Config File.vi"("Action"=enum16{"Write", "Read", "Read All", "Remove"}."Write", "file path"=w216, "error in (no error)"=w217, "Value"=w236, "Key Name"=w235, "TestPlan Section"="Log VL" ("TestPlan Name")) -> ("error out"=w215:errorcluster)  [unwired: 3 in, 2 out]
              }
              event "Sub Log": Value Change {
                n94 = event-data() -> ()  [unwired: 1 in, 1 out]
                n95 = To Unsigned Byte Integer(number="Sub Log") -> (unsigned 8bit integer=w243:u8)
                n96 = local write "LOG Table"(w243) -> ()
              }
              event "Start Enable": Value Change {
                n97 = event-data() -> ("NewVal"=w250:bool)  [unwired: 1 in]
                n98 = Select(t=T7."Enabled" ("Disabled"), s=w250, f=T7."Disabled and Grayed Out") -> (s? t:f=w248:T7)
                n99 = property on="Start Tab" class="TabCtl (strict)"(error in=w252, "DisabledEnum"=w248) -> (error out=w253:errorcluster)  [unwired: 1 in, 1 out]
              }
              event "Stop Enable": Value Change {
                n100 = event-data() -> ("NewVal"=w260:bool)  [unwired: 1 in]
                n101 = Select(t=T7."Enabled" ("Disabled"), s=w260, f=T7."Disabled and Grayed Out") -> (s? t:f=w257:T7)
                n102 = property on="Stop Tab" class="TabCtl (strict)"(error in=w258, "DisabledEnum"=w257) -> (error out=w259:errorcluster)  [unwired: 1 in, 1 out]
              }
            }
          }
          frame "Load VL" {
            n103 = Empty String/Path?(string/path=w268) -> (empty?=w267:bool)
            n104 = case shown="False" w267 {
              tunnel: w269 -> [w279 w290]
              tunnel: [w272 w290] -> w264
              tunnel: w268 -> [_ _]
              tunnel: [w278 w289] -> w266
              tunnel: w265 -> [w278 w289]
              frame False {
                n105 = call "TestPlan - Config File.vi"("Action"=enum16{"Write", "Read", "Read All", "Remove"}."Read", "file path"=w278, "error in (no error)"=w279, "TestPlan Section"="Log VL" ("TestPlan Name")) -> ("error out"=w275:errorcluster, "key names"=w277:string[])  [unwired: 5 in, 1 out]
                n106 = for {
                  tunnel: w277 -> [w288] mode=indexing
                  shift-right: [w287] -> w276
                  shift-left: w275 -> [w287]
                  tunnel: [w285] -> w274 mode=indexing
                  n107 = Match Pattern(string=w288, regular expression="-") -> (before substring=w285:string)  [unwired: 1 in, 3 out]
                }
                n108 = call "TestPlan - Remove Duplicate.vi"("Input Array"=w274) -> ("Output Array"=w273:string[])  [unwired: 1 out]
                n109 = Build Array (concatenate)("Please select", w273) -> (w284:string[])
                n110 = property on="Log VL" class="Ring (strict)"(error in=w276, "Strings []"=w284) -> (error out=w283:errorcluster)  [unwired: 1 in, 1 out]
                n111 = call <vilib>:"Clear Errors.vi"("error in (no error)"=w283, "specific error code to clear (0: all)"=7) -> ("error out"=w272:errorcluster)  [unwired: 4 in, 1 out]
              }
              frame True {
              }
            }
          }
          frame "Load Start" {
            n112 = Empty String/Path?(string/path=w295) -> (empty?=w294:bool)
            n113 = case shown="False" w294 {
              tunnel: w296 -> [w305 w460]
              tunnel: [w300 w462] -> w291
              tunnel: w295 -> [_ _]
              tunnel: [w304 w463] -> w293
              tunnel: w292 -> [w304 w463]
              frame False {
                n114 = call "TestPlan - Config File.vi"("Action"=enum16{"Write", "Read", "Read All", "Remove"}."Read", "file path"=w304, "error in (no error)"=w305, "TestPlan Section"="Start Condition" ("TestPlan Name")) -> ("error out"=w298:errorcluster, "Value Out"=w302:T8)  [unwired: 5 in, 1 out]
                n115 = Index Array(array=w302) -> (element=w301:T9)  [unwired: 1 in]
                n116 = Unbundle By Name(w301) -> ("Key Value"=w299:string[])
                n117 = for {
                  shift-right: [w307] -> w300
                  shift-left: w298 -> [w309]
                  tunnel: w299 -> [w308] mode=indexing
                  i -> [w310]
                  n118 = case shown="0, Default" w310 {
                    tunnel: w309 -> [w318 w331 w342 w362 w387 w409 w428 w439 w450]
                    tunnel: w308 -> [w316 w334 w341 w361 w386 w408 w427 w438 w449]
                    tunnel: [w315 w332 w342 w362 w387 w409 w428 w439 w450] -> w307
                    frame 0, Default {
                      n119 = property on="Test Type" class="Ring (strict)"(error in=w318) -> (error out=w315:errorcluster, "Strings []"=w317:string[])  [unwired: 1 in, 1 out]
                      n120 = Search 1D Array(1D array=w317, element=w316) -> (index of element=w311:i32)  [unwired: 1 in]
                      n121 = case shown="10" w311 {
                        tunnel: [w319 w320 w321 w322 w323 w324 w325 w326 w327 w328 w329] -> w314
                        tunnel: [w319 w320 w321 w322 w323 w324 w325 w326 w327 w328 w329] -> w313
                        tunnel: [w319 w320 w321 w322 w323 w324 w325 w326 w327 w328 w329] -> w312
                        frame 1 {
                          w319 = Test_Plan_-_Log_Conditions_Tab."TS" ("Log Tab")
                        }
                        frame 2 {
                          w320 = Test_Plan_-_Log_Conditions_Tab."TUU" ("Log Tab")
                        }
                        frame 3 {
                          w321 = Test_Plan_-_Log_Conditions_Tab."Shearbox" ("Log Tab")
                        }
                        frame 4 {
                          w322 = Test_Plan_-_Log_Conditions_Tab."Permiability" ("Log Tab")
                        }
                        frame 5 {
                          w323 = Test_Plan_-_Log_Conditions_Tab."Consolidation" ("Log Tab")
                        }
                        frame 6 {
                          w324 = Test_Plan_-_Log_Conditions_Tab."Saturation" ("Log Tab")
                        }
                        frame 7 {
                          w325 = Test_Plan_-_Log_Conditions_Tab."User Defined" ("Log Tab")
                        }
                        frame 8 {
                          w326 = Test_Plan_-_Log_Conditions_Tab."UCT" ("Log Tab")
                        }
                        frame 9 {
                          w327 = Test_Plan_-_Log_Conditions_Tab."Iso Consolidation" ("Log Tab")
                        }
                        frame 10 {
                          w328 = Test_Plan_-_Log_Conditions_Tab."SP" ("Log Tab")
                        }
                        frame Default {
                          w329 = Test_Plan_-_Log_Conditions_Tab."Others" ("Log Tab")
                        }
                      }
                      n122 = local write "Test Type"(w311) -> ()
                      n123 = local write "Log Tab"(w314) -> ()
                      n124 = local write "Start Tab"(w313) -> ()
                      n125 = local write "Stop Tab"(w312) -> ()
                    }
                    frame 1 {
                      # "Start Tab"
                      n126 = Equal?(x=w334, y="Disabled") -> (x = y?=w330:bool)
                      n127 = case shown="True" w330 {
                        tunnel: [w335 w338] -> w332
                        tunnel: w331 -> [w335 w337]
                        frame False {
                        }
                        frame True {
                          n128 = local write "Start Enable"(FALSE ("Start Enable")) -> ()
                          n129 = property on="Start Tab" class="TabCtl (strict)"(error in=w337, "DisabledEnum"=T7."Disabled and Grayed Out" ("Disabled")) -> (error out=w338:errorcluster)  [unwired: 1 in, 1 out]
                        }
                      }
                    }
                    frame 2 {
                      # "Test Type"
                      n130 = local read "Start Tab"() -> (w340:T3)
                      n131 = case shown="\"SP\"" w340 {
                        tunnel: w341 -> [_ w345 w347 w349 w351 w353 w355 w357 w359 _]
                        frame Default {
                        }
                        frame "Consolidation" {
                          n132 = Fract/Exp String To Number(string=w345, default (0 dbl)=0.0 ("Start Delay")) -> (number=w343:dbl)  [unwired: 2 in, 1 out]
                          n133 = local write "Cons Start VS"(w343) -> ()
                        }
                        frame "Saturation" {
                          n134 = Fract/Exp String To Number(string=w347) -> (number=w346:dbl)  [unwired: 3 in, 1 out]
                          n135 = local write "Sat CP"(w346) -> ()
                        }
                        frame "Iso Consolidation" {
                          n136 = Fract/Exp String To Number(string=w349) -> (number=w348:dbl)  [unwired: 3 in, 1 out]
                          n137 = local write "Iso BP"(w348) -> ()
                        }
                        frame "TS" {
                          n138 = Fract/Exp String To Number(string=w351) -> (number=w350:dbl)  [unwired: 3 in, 1 out]
                          n139 = local write "TS Shear Speed"(w350) -> ()
                        }
                        frame "TUU" {
                          n140 = Fract/Exp String To Number(string=w353) -> (number=w352:dbl)  [unwired: 3 in, 1 out]
                          n141 = local write "TUU Shear Speed"(w352) -> ()
                        }
                        frame "Shearbox" {
                          n142 = Fract/Exp String To Number(string=w355) -> (number=w354:dbl)  [unwired: 3 in, 1 out]
                          n143 = local write "SB Shear Speed"(w354) -> ()
                        }
                        frame "UCT" {
                          n144 = Fract/Exp String To Number(string=w357) -> (number=w356:dbl)  [unwired: 3 in, 1 out]
                          n145 = local write "UCT Shear Speed"(w356) -> ()
                        }
                        frame "Permiability" {
                          n146 = Fract/Exp String To Number(string=w359) -> (number=w358:dbl)  [unwired: 3 in, 1 out]
                          n147 = local write "Perm DP"(w358) -> ()
                        }
                        frame "SP" {
                        }
                      }
                    }
                    frame 3 {
                      # "Test Type"
                      n148 = local read "Start Tab"() -> (w360:T3)
                      n149 = case shown="\"Shearbox\"" w360 {
                        tunnel: w361 -> [_ w366 w370 w374 w378 w382 w384 _]
                        frame Default {
                        }
                        frame "Consolidation" {
                          n150 = Decimal String To Number(string=w366, default (0L)=u16 0 ("Start Delay")) -> (number=w364:u16)  [unwired: 1 in, 1 out]
                          n151 = Greater Than 0?(x=w364) -> (x > 0?=w363:bool)
                          n152 = local write "Cons Start .Delay"(w363) -> ()
                        }
                        frame "TS" {
                          n153 = Decimal String To Number(string=w370, default (0L)=u16 0 ("Start Delay")) -> (number=w368:u16)  [unwired: 1 in, 1 out]
                          n154 = Greater Than 0?(x=w368) -> (x > 0?=w367:bool)
                          n155 = local write "TS Engage"(w367) -> ()
                        }
                        frame "TUU" {
                          n156 = Decimal String To Number(string=w374, default (0L)=u16 0 ("Start Delay")) -> (number=w372:u16)  [unwired: 1 in, 1 out]
                          n157 = Greater Than 0?(x=w372) -> (x > 0?=w371:bool)
                          n158 = local write "TUU Engage"(w371) -> ()
                        }
                        frame "Shearbox" {
                          n159 = Decimal String To Number(string=w378, default (0L)=u16 0 ("Start Delay")) -> (number=w376:u16)  [unwired: 1 in, 1 out]
                          n160 = Greater Than 0?(x=w376) -> (x > 0?=w375:bool)
                          n161 = local write "SB Engage"(w375) -> ()
                        }
                        frame "UCT" {
                          n162 = Decimal String To Number(string=w382, default (0L)=u16 0 ("Start Delay")) -> (number=w380:u16)  [unwired: 1 in, 1 out]
                          n163 = Greater Than 0?(x=w380) -> (x > 0?=w379:bool)
                          n164 = local write "UCT Engage"(w379) -> ()
                        }
                        frame "Saturation" {
                          n165 = Fract/Exp String To Number(string=w384) -> (number=w383:dbl)  [unwired: 3 in, 1 out]
                          n166 = local write "Sat BP"(w383) -> ()
                        }
                        frame "Iso Consolidation" {
                        }
                      }
                    }
                    frame 4 {
                      # "Test Type"
                      n167 = local read "Start Tab"() -> (w385:T3)
                      n168 = case shown="\"Shearbox\"" w385 {
                        tunnel: w386 -> [_ w391 w394 _ w397 w400 w403 w406]
                        frame Default {
                        }
                        frame "Consolidation" {
                          n169 = Fract/Exp String To Number(string=w391, default (0 dbl)=0.0 ("Start Delay")) -> (number=w389:dbl)  [unwired: 2 in, 1 out]
                          n170 = call "Main - Seconds to Time (SubVI).vi"("Seconds"=w389) -> ("Time"=w388:timestamp)  [unwired: 9 in, 1 out]
                          n171 = local write "Cons Start Delay"(w388) -> ()
                        }
                        frame "Saturation" {
                          n172 = Decimal String To Number(string=w394) -> (number=w393:i32)  [unwired: 2 in, 1 out]
                          n173 = Greater Than 0?(x=w393) -> (x > 0?=w392:bool)
                          n174 = local write "Sat Start BP"(w392) -> ()
                        }
                        frame "Iso Consolidation" {
                        }
                        frame "TS" {
                          n175 = Fract/Exp String To Number(string=w397, default (0 dbl)=0.0 ("Start Delay")) -> (number=w395:dbl)  [unwired: 2 in, 1 out]
                          n176 = local write "TS Engage Speed"(w395) -> ()
                        }
                        frame "TUU" {
                          n177 = Fract/Exp String To Number(string=w400, default (0 dbl)=0.0 ("Start Delay")) -> (number=w398:dbl)  [unwired: 2 in, 1 out]
                          n178 = local write "TUU Engage Speed"(w398) -> ()
                        }
                        frame "Shearbox" {
                          n179 = Fract/Exp String To Number(string=w403, default (0 dbl)=0.0 ("Start Delay")) -> (number=w401:dbl)  [unwired: 2 in, 1 out]
                          n180 = local write "SB Engage Speed"(w401) -> ()
                        }
                        frame "UCT" {
                          n181 = Fract/Exp String To Number(string=w406, default (0 dbl)=0.0 ("Start Delay")) -> (number=w404:dbl)  [unwired: 2 in, 1 out]
                          n182 = local write "UCT Engage Speed"(w404) -> ()
                        }
                      }
                    }
                    frame 5 {
                      # "Test Type"
                      n183 = local read "Start Tab"() -> (w407:T3)
                      n184 = case shown="\"Shearbox\"" w407 {
                        tunnel: w408 -> [_ w413 _ _ w416 w419 w422 w425]
                        frame Default {
                        }
                        frame "Consolidation" {
                          n185 = Fract/Exp String To Number(string=w413, default (0 dbl)=0.0 ("Start Delay")) -> (number=w411:dbl)  [unwired: 2 in, 1 out]
                          n186 = call "Main - Seconds to Time (SubVI).vi"("Seconds"=w411) -> ("Time"=w410:timestamp)  [unwired: 9 in, 1 out]
                          n187 = local write "Cons Start Delay"(w410) -> ()
                        }
                        frame "Saturation" {
                        }
                        frame "Iso Consolidation" {
                        }
                        frame "TS" {
                          n188 = Fract/Exp String To Number(string=w416, default (0 dbl)=0.0 ("Start Delay")) -> (number=w414:dbl)  [unwired: 2 in, 1 out]
                          n189 = local write "TS Load Change"(w414) -> ()
                        }
                        frame "TUU" {
                          n190 = Fract/Exp String To Number(string=w419, default (0 dbl)=0.0 ("Start Delay")) -> (number=w417:dbl)  [unwired: 2 in, 1 out]
                          n191 = local write "TUU Load Change"(w417) -> ()
                        }
                        frame "Shearbox" {
                          n192 = Fract/Exp String To Number(string=w422, default (0 dbl)=0.0 ("Start Delay")) -> (number=w420:dbl)  [unwired: 2 in, 1 out]
                          n193 = local write "SB Load Change"(w420) -> ()
                        }
                        frame "UCT" {
                          n194 = Fract/Exp String To Number(string=w425, default (0 dbl)=0.0 ("Start Delay")) -> (number=w423:dbl)  [unwired: 2 in, 1 out]
                          n195 = local write "UCT Load Change"(w423) -> ()
                        }
                      }
                    }
                    frame 6 {
                      # "Test Type"
                      n196 = local read "Start Tab"() -> (w426:T3)
                      n197 = case shown="\"Shearbox\"" w426 {
                        tunnel: w427 -> [_ w430 w433 w436]
                        frame Default {
                        }
                        frame "TS" {
                          n198 = Decimal String To Number(string=w430) -> (number=w429:i32)  [unwired: 2 in, 1 out]
                          n199 = local write "TS Drain"(w429) -> ()
                        }
                        frame "TUU" {
                          n200 = Fract/Exp String To Number(string=w433, default (0 dbl)=0.0 ("Start Delay")) -> (number=w431:dbl)  [unwired: 2 in, 1 out]
                          n201 = local write "TUU Confining Pressure"(w431) -> ()
                        }
                        frame "Shearbox" {
                          n202 = Fract/Exp String To Number(string=w436, default (0 dbl)=0.0 ("Start Delay")) -> (number=w434:dbl)  [unwired: 2 in, 1 out]
                          n203 = local write "SB Vertical Load"(w434) -> ()
                        }
                      }
                    }
                    frame 8 {
                      # "Test Type"
                      n204 = local read "Start Tab"() -> (w437:T3)
                      n205 = case shown="\"Shearbox\"" w437 {
                        tunnel: w438 -> [_ w443 w447]
                        frame Default {
                        }
                        frame "TUU" {
                          n206 = Fract/Exp String To Number(string=w443, default (0 dbl)=0.0 ("Start Delay")) -> (number=w441:dbl)  [unwired: 2 in, 1 out]
                          n207 = call "Main - Seconds to Time (SubVI).vi"("Seconds"=w441) -> ("Time"=w440:timestamp)  [unwired: 9 in, 1 out]
                          n208 = local write "TUU Start Delay"(w440) -> ()
                        }
                        frame "Shearbox" {
                          n209 = Fract/Exp String To Number(string=w447, default (0 dbl)=0.0 ("Start Delay")) -> (number=w445:dbl)  [unwired: 2 in, 1 out]
                          n210 = call "Main - Seconds to Time (SubVI).vi"("Seconds"=w445) -> ("Time"=w444:timestamp)  [unwired: 9 in, 1 out]
                          n211 = local write "SB Start Delay"(w444) -> ()
                        }
                      }
                    }
                    frame 7 {
                      # "Test Type"
                      n212 = local read "Start Tab"() -> (w448:T3)
                      n213 = case shown="\"Shearbox\"" w448 {
                        tunnel: w449 -> [_ w452 w456]
                        frame Default {
                        }
                        frame "TUU" {
                          n214 = Decimal String To Number(string=w452, default (0L)=u16 0 ("Start Delay")) -> (number=w453:u16)  [unwired: 1 in, 1 out]
                          n215 = Greater Than 0?(x=w453) -> (x > 0?=w451:bool)
                          n216 = local write "TUU Start .Delay"(w451) -> ()
                        }
                        frame "Shearbox" {
                          n217 = Decimal String To Number(string=w456, default (0L)=u16 0 ("Start Delay")) -> (number=w457:u16)  [unwired: 1 in, 1 out]
                          n218 = Greater Than 0?(x=w457) -> (x > 0?=w455:bool)
                          n219 = local write "SB Start .Delay"(w455) -> ()
                        }
                      }
                    }
                  }
                }
              }
              frame True {
                n220 = property on="Test Type" class="Ring (strict)"(error in=w460) -> (error out=w461:errorcluster, "Strings []"=w459:string[])  [unwired: 1 in, 1 out]
                n221 = for {
                  shift-right: [w466] -> w462
                  shift-left: w461 -> [w465]
                  tunnel: w459 -> [_] mode=indexing
                  i -> [w464]
                  n222 = case shown="0, Default" w464 {
                    tunnel: [w467 w468] -> w466
                    tunnel: w465 -> [w467 w468]
                    frame 0, Default {
                    }
                    frame 5 {
                      n223 = local write "Cons Stop Select"(enum32{"1", "2", "3"}."1" ("Cons Stop Select")) -> ()
                      n224 = local write "Cons Log Select"(enum32{"1", "2"}."1" ("Cons Log Select")) -> ()
                    }
                  }
                }
              }
            }
          }
          frame "Load Log" {
            n225 = Empty String/Path?(string/path=w475) -> (empty?=w474:bool)
            n226 = case shown="False" w474 {
              tunnel: w476 -> [w485 w788]
              tunnel: [w480 w788] -> w471
              tunnel: w475 -> [_ _]
              tunnel: [w484 w787] -> w473
              tunnel: w472 -> [w484 w787]
              frame False {
                n227 = call "TestPlan - Config File.vi"("Action"=enum16{"Write", "Read", "Read All", "Remove"}."Read", "file path"=w484, "error in (no error)"=w485, "TestPlan Section"="Log Condition" ("TestPlan Name")) -> ("error out"=w478:errorcluster, "Value Out"=w482:T8)  [unwired: 5 in, 1 out]
                n228 = Index Array(array=w482) -> (element=w481:T9)  [unwired: 1 in]
                n229 = Unbundle By Name(w481) -> ("Key Value"=w479:string[])
                n230 = for {
                  shift-right: [w489] -> w480
                  shift-left: w478 -> [w491]
                  tunnel: w479 -> [w490] mode=indexing
                  shift-right: [w488] -> _
                  shift-left: _ -> [w487]
                  i -> [w492]
                  n231 = case shown="3" w492 {
                    tunnel: w491 -> [w494 w500 w524 w574 w676 w776]
                    tunnel: w490 -> [_ w499 w528 w573 w675 w775]
                    tunnel: [w494 w500 w525 w575 w677 w776] -> w489
                    tunnel: w487 -> [_ w496 w523 w568 w670 w772]
                    tunnel: [w493 w495 w522 w567 w669 w771] -> w488
                    frame 0, Default {
                      # "test type already load"
                      n232 = local read "Log Tab"() -> (w493:T4)
                    }
                    frame 1 {
                      n233 = Decimal String To Number(string=w499, default (0L)=u16 0 ("Start Delay")) -> (number=w497:u16)  [unwired: 1 in, 1 out]
                      n234 = case shown="\"SP\"" w496 {
                        selector: w496 -> [w501 w503 w505 w507 w509 w512 w515 w518 w520 w521]
                        tunnel: w497 -> [_ w502 w504 w506 w508 w511 w514 w517 _ _]
                        tunnel: [w501 w503 w505 w507 w509 w512 w515 w518 w520 w521] -> w495
                        frame Default {
                        }
                        frame "Consolidation" {
                          n235 = local write "ConsTable"(w502) -> ()
                          n236 = local write "Cons Log Select"(w502) -> ()
                        }
                        frame "Saturation" {
                          n237 = local write "Sat Log Select"(w504) -> ()
                          n238 = local write "SatTable"(w504) -> ()
                        }
                        frame "Iso Consolidation" {
                          n239 = local write "IsoTable"(w506) -> ()
                          n240 = local write "Iso Log Select"(w506) -> ()
                        }
                        frame "TS" {
                          n241 = case shown="1" w508 {
                            frame 0, Default {
                            }
                            frame 1 {
                              n242 = local write "TSTable"(enum32{"None", "Time", "Disp"}."Disp" ("TSTable")) -> ()
                            }
                          }
                          n243 = local write "TS Log Select"(w508) -> ()
                        }
                        frame "TUU" {
                          n244 = case shown="1" w511 {
                            frame 0, Default {
                            }
                            frame 1 {
                              n245 = local write "TUUTable"(enum32{"None", "Time", "Disp"}."Disp" ("TUUTable")) -> ()
                            }
                          }
                          n246 = local write "TUU Log Select"(w511) -> ()
                        }
                        frame "Shearbox" {
                          n247 = case shown="1" w514 {
                            frame 0, Default {
                            }
                            frame 1 {
                              n248 = local write "SBTable"(enum32{"None", "Time", "Disp"}."Disp" ("TUUTable")) -> ()
                            }
                          }
                          n249 = local write "SB Log Select"(w514) -> ()
                        }
                        frame "UCT" {
                          n250 = case shown="1" w517 {
                            frame 0, Default {
                            }
                            frame 1 {
                              n251 = local write "UCTTable"(enum32{"None", "Time", "Disp"}."Disp" ("UCTTable")) -> ()
                            }
                          }
                          n252 = local write "UCT Log Select"(w517) -> ()
                        }
                        frame "Permiability" {
                        }
                        frame "SP" {
                        }
                      }
                    }
                    frame 2 {
                      n253 = Decimal String To Number(string=w528, default (0L)=0.0 ("Start Delay")) -> (number=w526:dbl)  [unwired: 1 in, 1 out]
                      n254 = case shown="\"SP\"" w523 {
                        selector: w523 -> [w529 w531 w535 w539 w544 w548 w552 w556 w560 w564]
                        tunnel: w526 -> [_ w533 w537 w541 w545 w549 w553 w557 w561 w565]
                        tunnel: [w530 w534 w538 w542 w546 w550 w554 w558 w562 w566] -> w525
                        tunnel: w524 -> [w530 w534 w538 w542 w546 w550 w554 w558 w562 w566]
                        tunnel: [w529 w531 w535 w539 w544 w548 w552 w556 w560 w564] -> w522
                        frame Default {
                        }
                        frame "Consolidation" {
                          n255 = call "Main - Seconds to Time (SubVI).vi"("Seconds"=w533) -> ("Time"=w532:timestamp)  [unwired: 9 in, 1 out]
                          n256 = local write "Cons Log Delay"(w532) -> ()
                        }
                        frame "Saturation" {
                          n257 = call "Main - Seconds to Time (SubVI).vi"("Seconds"=w537) -> ("Time"=w536:timestamp)  [unwired: 9 in, 1 out]
                          n258 = local write "Sat Log Delay"(w536) -> ()
                        }
                        frame "Iso Consolidation" {
                          n259 = call "Main - Seconds to Time (SubVI).vi"("Seconds"=w541) -> ("Time"=w540:timestamp)  [unwired: 9 in, 1 out]
                          n260 = local write "Iso Log Delay"(w540) -> ()
                        }
                        frame "TS" {
                          n261 = call "Main - Seconds to Time (SubVI).vi"("Seconds"=w545) -> ("Time"=w543:timestamp)  [unwired: 9 in, 1 out]
                          n262 = local write "TS Log Delay"(w543) -> ()
                        }
                        frame "TUU" {
                          n263 = call "Main - Seconds to Time (SubVI).vi"("Seconds"=w549) -> ("Time"=w547:timestamp)  [unwired: 9 in, 1 out]
                          n264 = local write "TUU Log Delay"(w547) -> ()
                        }
                        frame "Shearbox" {
                          n265 = call "Main - Seconds to Time (SubVI).vi"("Seconds"=w553) -> ("Time"=w551:timestamp)  [unwired: 9 in, 1 out]
                          n266 = local write "SB Log Delay"(w551) -> ()
                        }
                        frame "Permiability" {
                          n267 = call "Main - Seconds to Time (SubVI).vi"("Seconds"=w557) -> ("Time"=w555:timestamp)  [unwired: 9 in, 1 out]
                          n268 = local write "Perm Log Delay"(w555) -> ()
                        }
                        frame "SP" {
                          n269 = call "Main - Seconds to Time (SubVI).vi"("Seconds"=w561) -> ("Time"=w559:timestamp)  [unwired: 9 in, 1 out]
                          n270 = local write "SP Log Delay"(w559) -> ()
                        }
                        frame "UCT" {
                          n271 = call "Main - Seconds to Time (SubVI).vi"("Seconds"=w565) -> ("Time"=w563:timestamp)  [unwired: 9 in, 1 out]
                          n272 = local write "UCT Log Delay"(w563) -> ()
                        }
                      }
                    }
                    frame 3 {
                      n273 = Spreadsheet String To Array(delimiter (Tab)=",", format string="", spreadsheet string=w573, array type (2D Dbl)=string[] []) -> (array=w571:string[])
                      n274 = case shown="\"Shearbox\"" w568 {
                        selector: w568 -> [w576 w578 w591 w604 w618 w631 w644 w657]
                        tunnel: [w577 w580 w593 w606 w619 w632 w645 w658] -> w575
                        tunnel: w574 -> [w577 w581 w594 w607 w620 w633 w646 w659]
                        tunnel: w571 -> [_ w582 w595 w608 w621 w634 w647 w660]
                        tunnel: [w576 w578 w591 w604 w618 w631 w644 w657] -> w567
                        frame Default {
                        }
                        frame "Consolidation" {
                          n275 = for {
                            tunnel: w582 -> [w585] mode=indexing
                            shift-right: [w588] -> w580
                            shift-left: w581 -> [w589]
                            tunnel: [w583] -> w579 mode=indexing
                            i -> [w587]
                            n276 = Increment(x=w587) -> (x+1=w586:i32)
                            n277 = Format Into String(format string="%d", error in=w589, w586) -> (resulting string=w584:string, error out=w588:errorcluster)  [unwired: 1 in]
                            n278 = Build Array(w584, w585) -> (w583:string[])
                          }
                          n279 = local write "Cons LogTime"(w579) -> ()
                        }
                        frame "Saturation" {
                          n280 = for {
                            tunnel: w595 -> [w598] mode=indexing
                            shift-right: [w601] -> w593
                            shift-left: w594 -> [w602]
                            tunnel: [w596] -> w592 mode=indexing
                            i -> [w600]
                            n281 = Increment(x=w600) -> (x+1=w599:i32)
                            n282 = Format Into String(format string="%d", error in=w602, w599) -> (resulting string=w597:string, error out=w601:errorcluster)  [unwired: 1 in]
                            n283 = Build Array(w597, w598) -> (w596:string[])
                          }
                          n284 = local write "Sat LogTime"(w592) -> ()
                        }
                        frame "Iso Consolidation" {
                          n285 = for {
                            tunnel: w608 -> [w611] mode=indexing
                            shift-right: [w614] -> w606
                            shift-left: w607 -> [w615]
                            tunnel: [w609] -> w605 mode=indexing
                            i -> [w613]
                            n286 = Increment(x=w613) -> (x+1=w612:i32)
                            n287 = Format Into String(format string="%d", error in=w615, w612) -> (resulting string=w610:string, error out=w614:errorcluster)  [unwired: 1 in]
                            n288 = Build Array(w610, w611) -> (w609:string[])
                          }
                          n289 = local write "Iso LogTime"(w605) -> ()
                        }
                        frame "TS" {
                          n290 = for {
                            tunnel: w621 -> [w624] mode=indexing
                            shift-right: [w627] -> w619
                            shift-left: w620 -> [w628]
                            tunnel: [w622] -> w617 mode=indexing
                            i -> [w626]
                            n291 = Increment(x=w626) -> (x+1=w625:i32)
                            n292 = Format Into String(format string="%d", error in=w628, w625) -> (resulting string=w623:string, error out=w627:errorcluster)  [unwired: 1 in]
                            n293 = Build Array(w623, w624) -> (w622:string[])
                          }
                          n294 = local write "TS LogTime"(w617) -> ()
                        }
                        frame "TUU" {
                          n295 = for {
                            tunnel: w634 -> [w637] mode=indexing
                            shift-right: [w640] -> w632
                            shift-left: w633 -> [w641]
                            tunnel: [w635] -> w630 mode=indexing
                            i -> [w639]
                            n296 = Increment(x=w639) -> (x+1=w638:i32)
                            n297 = Format Into String(format string="%d", error in=w641, w638) -> (resulting string=w636:string, error out=w640:errorcluster)  [unwired: 1 in]
                            n298 = Build Array(w636, w637) -> (w635:string[])
                          }
                          n299 = local write "TUU LogTime"(w630) -> ()
                        }
                        frame "Shearbox" {
                          n300 = for {
                            tunnel: w647 -> [w650] mode=indexing
                            shift-right: [w653] -> w645
                            shift-left: w646 -> [w654]
                            tunnel: [w648] -> w643 mode=indexing
                            i -> [w652]
                            n301 = Increment(x=w652) -> (x+1=w651:i32)
                            n302 = Format Into String(format string="%d", error in=w654, w651) -> (resulting string=w649:string, error out=w653:errorcluster)  [unwired: 1 in]
                            n303 = Build Array(w649, w650) -> (w648:string[])
                          }
                          n304 = local write "SB LogTime"(w643) -> ()
                        }
                        frame "UCT" {
                          n305 = for {
                            tunnel: w660 -> [w663] mode=indexing
                            shift-right: [w666] -> w658
                            shift-left: w659 -> [w667]
                            tunnel: [w661] -> w656 mode=indexing
                            i -> [w665]
                            n306 = Increment(x=w665) -> (x+1=w664:i32)
                            n307 = Format Into String(format string="%d", error in=w667, w664) -> (resulting string=w662:string, error out=w666:errorcluster)  [unwired: 1 in]
                            n308 = Build Array(w662, w663) -> (w661:string[])
                          }
                          n309 = local write "UCT LogTime"(w656) -> ()
                        }
                      }
                    }
                    frame 4 {
                      n310 = Spreadsheet String To Array(delimiter (Tab)=",", format string="", spreadsheet string=w675, array type (2D Dbl)=string[] []) -> (array=w673:string[])
                      n311 = case shown="\"Shearbox\"" w670 {
                        selector: w670 -> [w678 w680 w693 w706 w720 w733 w746 w759]
                        tunnel: [w679 w682 w695 w708 w721 w734 w747 w760] -> w677
                        tunnel: w676 -> [w679 w683 w696 w709 w722 w735 w748 w761]
                        tunnel: w673 -> [_ w684 w697 w710 w723 w736 w749 w762]
                        tunnel: [w678 w680 w693 w706 w720 w733 w746 w759] -> w669
                        frame Default {
                        }
                        frame "Consolidation" {
                          n312 = for {
                            tunnel: w684 -> [w687] mode=indexing
                            shift-right: [w690] -> w682
                            shift-left: w683 -> [w691]
                            tunnel: [w685] -> w681 mode=indexing
                            i -> [w689]
                            n313 = Increment(x=w689) -> (x+1=w688:i32)
                            n314 = Format Into String(format string="%d", error in=w691, w688) -> (resulting string=w686:string, error out=w690:errorcluster)  [unwired: 1 in]
                            n315 = Build Array(w686, w687) -> (w685:string[])
                          }
                          n316 = local write "Cons LogDisp"(w681) -> ()
                        }
                        frame "Saturation" {
                          n317 = for {
                            tunnel: w697 -> [w700] mode=indexing
                            shift-right: [w703] -> w695
                            shift-left: w696 -> [w704]
                            tunnel: [w698] -> w694 mode=indexing
                            i -> [w702]
                            n318 = Increment(x=w702) -> (x+1=w701:i32)
                            n319 = Format Into String(format string="%d", error in=w704, w701) -> (resulting string=w699:string, error out=w703:errorcluster)  [unwired: 1 in]
                            n320 = Build Array(w699, w700) -> (w698:string[])
                          }
                          n321 = local write "Sat LogDisp"(w694) -> ()
                        }
                        frame "Iso Consolidation" {
                          n322 = for {
                            tunnel: w710 -> [w713] mode=indexing
                            shift-right: [w716] -> w708
                            shift-left: w709 -> [w717]
                            tunnel: [w711] -> w707 mode=indexing
                            i -> [w715]
                            n323 = Increment(x=w715) -> (x+1=w714:i32)
                            n324 = Format Into String(format string="%d", error in=w717, w714) -> (resulting string=w712:string, error out=w716:errorcluster)  [unwired: 1 in]
                            n325 = Build Array(w712, w713) -> (w711:string[])
                          }
                          n326 = local write "Iso LogDisp"(w707) -> ()
                        }
                        frame "TS" {
                          n327 = for {
                            tunnel: w723 -> [w726] mode=indexing
                            shift-right: [w729] -> w721
                            shift-left: w722 -> [w730]
                            tunnel: [w724] -> w719 mode=indexing
                            i -> [w728]
                            n328 = Increment(x=w728) -> (x+1=w727:i32)
                            n329 = Format Into String(format string="%d", error in=w730, w727) -> (resulting string=w725:string, error out=w729:errorcluster)  [unwired: 1 in]
                            n330 = Build Array(w725, w726) -> (w724:string[])
                          }
                          n331 = local write "TS LogDisp"(w719) -> ()
                        }
                        frame "TUU" {
                          n332 = for {
                            tunnel: w736 -> [w739] mode=indexing
                            shift-right: [w742] -> w734
                            shift-left: w735 -> [w743]
                            tunnel: [w737] -> w732 mode=indexing
                            i -> [w741]
                            n333 = Increment(x=w741) -> (x+1=w740:i32)
                            n334 = Format Into String(format string="%d", error in=w743, w740) -> (resulting string=w738:string, error out=w742:errorcluster)  [unwired: 1 in]
                            n335 = Build Array(w738, w739) -> (w737:string[])
                          }
                          n336 = local write "TUU LogDisp"(w732) -> ()
                        }
                        frame "Shearbox" {
                          n337 = for {
                            tunnel: w749 -> [w752] mode=indexing
                            shift-right: [w755] -> w747
                            shift-left: w748 -> [w756]
                            tunnel: [w750] -> w745 mode=indexing
                            i -> [w754]
                            n338 = Increment(x=w754) -> (x+1=w753:i32)
                            n339 = Format Into String(format string="%d", error in=w756, w753) -> (resulting string=w751:string, error out=w755:errorcluster)  [unwired: 1 in]
                            n340 = Build Array(w751, w752) -> (w750:string[])
                          }
                          n341 = local write "SB LogDisp"(w745) -> ()
                        }
                        frame "UCT" {
                          n342 = for {
                            tunnel: w762 -> [w765] mode=indexing
                            shift-right: [w768] -> w760
                            shift-left: w761 -> [w769]
                            tunnel: [w763] -> w758 mode=indexing
                            i -> [w767]
                            n343 = Increment(x=w767) -> (x+1=w766:i32)
                            n344 = Format Into String(format string="%d", error in=w769, w766) -> (resulting string=w764:string, error out=w768:errorcluster)  [unwired: 1 in]
                            n345 = Build Array(w764, w765) -> (w763:string[])
                          }
                          n346 = local write "UCT LogDisp"(w758) -> ()
                        }
                      }
                    }
                    frame 5 {
                      n347 = Fract/Exp String To Number(string=w775, default (0 dbl)=sgl 0.0 ("Start Delay")) -> (number=w773:sgl)  [unwired: 2 in, 1 out]
                      n348 = case shown="\"TUU\"" w772 {
                        selector: w772 -> [w777 w778 w779 w780 w782 w784 w786]
                        tunnel: w773 -> [_ _ _ _ w781 w783 w785]
                        tunnel: [w777 w778 w779 w780 w782 w784 w786] -> w771
                        frame Default {
                        }
                        frame "Consolidation" {
                        }
                        frame "Saturation" {
                        }
                        frame "Iso Consolidation" {
                        }
                        frame "TS" {
                          n349 = local write "TS LogAxial"(w781) -> ()
                        }
                        frame "TUU" {
                          n350 = local write "TUU LogAxial"(w783) -> ()
                        }
                        frame "UCT" {
                          n351 = local write "UCT LogAxial"(w785) -> ()
                        }
                      }
                    }
                  }
                }
              }
              frame True {
              }
            }
          }
          frame "Load Stop" {
            n352 = Empty String/Path?(string/path=w793) -> (empty?=w792:bool)
            n353 = case shown="False" w792 {
              tunnel: w794 -> [w803 w1117]
              tunnel: [w798 w1117] -> w789
              tunnel: w793 -> [_ _]
              tunnel: [w802 w1116] -> w791
              tunnel: w790 -> [w802 w1116]
              frame False {
                n354 = call "TestPlan - Config File.vi"("Action"=enum16{"Write", "Read", "Read All", "Remove"}."Read", "file path"=w802, "error in (no error)"=w803, "TestPlan Section"="Stop Condition" ("TestPlan Name")) -> ("error out"=w796:errorcluster, "Value Out"=w800:T8)  [unwired: 5 in, 1 out]
                n355 = Index Array(array=w800) -> (element=w799:T9)  [unwired: 1 in]
                n356 = Unbundle By Name(w799) -> ("Key Value"=w797:string[])
                n357 = for {
                  shift-right: [w807] -> w798
                  shift-left: w796 -> [w809]
                  tunnel: w797 -> [w808] mode=indexing
                  shift-right: [w806] -> _
                  shift-left: _ -> [w805]
                  i -> [w810]
                  n358 = case shown="4" w810 {
                    tunnel: w809 -> [w812 w826 w842 w891 w936 w986 w1037 w1078 w1100]
                    tunnel: w808 -> [w815 w825 w839 w888 w933 w983 w1034 w1075 w1097]
                    tunnel: [w813 w826 w843 w892 w937 w987 w1038 w1079 w1101] -> w807
                    tunnel: [w816 w823 w840 w889 w934 w984 w1035 w1076 w1098] -> w806
                    tunnel: w805 -> [_ w823 w841 w890 w935 w985 w1036 w1077 w1099]
                    frame 0, Default {
                      # "test type already load"
                      n359 = Equal?(x=w815, y="Disabled") -> (x = y?=w811:bool)
                      n360 = case shown="False" w811 {
                        tunnel: [w817 w819] -> w813
                        tunnel: w812 -> [w817 w818]
                        frame False {
                        }
                        frame True {
                          n361 = local write "Stop Enable"(FALSE ("Stop Enable")) -> ()
                          n362 = property on="Stop Tab" class="TabCtl (strict)"(error in=w818, "DisabledEnum"=T7."Disabled and Grayed Out" ("Disabled")) -> (error out=w819:errorcluster)  [unwired: 1 in, 1 out]
                        }
                      }
                      n363 = local read "Stop Tab"() -> (w816:T5)
                    }
                    frame 1 {
                      n364 = Fract/Exp String To Number(string=w825, default (0 dbl)=0.0 ("Start Delay")) -> (number=w822:dbl)  [unwired: 2 in, 1 out]
                      n365 = case shown="\"UCT\"" w823 {
                        tunnel: w822 -> [w827 w828 w830 w831 w832 w833 w835 w837 w838]
                        frame "Consolidation", Default {
                          n366 = local write "Cons Stop Select"(w827) -> ()
                        }
                        frame "Saturation" {
                          n367 = local write "Sat Stop Select"(w828) -> ()
                        }
                        frame "Iso Consolidation" {
                          n368 = Greater Than 0?(x=w830) -> (x > 0?=w829:bool)
                          n369 = local write "Iso Stop .PP"(w829) -> ()
                        }
                        frame "TS" {
                          n370 = local write "TS Axial Value"(w831) -> ()
                        }
                        frame "TUU" {
                          n371 = local write "TUU Axial Value"(w832) -> ()
                        }
                        frame "Shearbox" {
                          n372 = local write "SB Shear Value"(w833) -> ()
                        }
                        frame "Permiability" {
                          n373 = call "Main - Seconds to Time (SubVI).vi"("Seconds"=w835) -> ("Time string"=w834:string)  [unwired: 9 in, 1 out]
                          n374 = local write "Perm Stop Time"(w834) -> ()
                        }
                        frame "SP" {
                          n375 = call "Main - Seconds to Time (SubVI).vi"("Seconds"=w837) -> ("Time string"=w836:string)  [unwired: 9 in, 1 out]
                          n376 = local write "SP Stop Time"(w836) -> ()
                        }
                        frame "UCT" {
                          n377 = local write "UCT Axial Value"(w838) -> ()
                        }
                      }
                    }
                    frame 2 {
                      n378 = case shown="\"UCT\"" w841 {
                        selector: w841 -> [w844 w848 w852 w856 w861 w866 w871 w876 w881 w886]
                        tunnel: [w845 w849 w853 w857 w862 w867 w872 w877 w882 w887] -> w843
                        tunnel: w842 -> [w845 w849 w853 w857 w862 w867 w872 w877 w882 w887]
                        tunnel: [w844 w848 w852 w856 w861 w866 w871 w876 w881 w886] -> w840
                        tunnel: w839 -> [_ w847 w851 w855 w860 w865 w870 w875 w880 w885]
                        frame Default {
                        }
                        frame "Consolidation" {
                          n379 = Fract/Exp String To Number(string=w847) -> (number=w846:dbl)  [unwired: 3 in, 1 out]
                          n380 = local write "Cons Stop Disp"(w846) -> ()
                        }
                        frame "Saturation" {
                          n381 = Fract/Exp String To Number(string=w851) -> (number=w850:dbl)  [unwired: 3 in, 1 out]
                          n382 = local write "Sat Stop PP"(w850) -> ()
                        }
                        frame "Iso Consolidation" {
                          n383 = Decimal String To Number(string=w855) -> (number=w854:i32)  [unwired: 2 in, 1 out]
                          n384 = local write "Iso Stop Select"(w854) -> ()
                        }
                        frame "TS" {
                          n385 = Decimal String To Number(string=w860) -> (number=w859:i32)  [unwired: 2 in, 1 out]
                          n386 = Greater Than 0?(x=w859) -> (x > 0?=w858:bool)
                          n387 = local write "TS MaxDev"(w858) -> ()
                        }
                        frame "TUU" {
                          n388 = Decimal String To Number(string=w865) -> (number=w864:i32)  [unwired: 2 in, 1 out]
                          n389 = Greater Than 0?(x=w864) -> (x > 0?=w863:bool)
                          n390 = local write "TUU MaxDev"(w863) -> ()
                        }
                        frame "Shearbox" {
                          n391 = Decimal String To Number(string=w870) -> (number=w869:i32)  [unwired: 2 in, 1 out]
                          n392 = Greater Than 0?(x=w869) -> (x > 0?=w868:bool)
                          n393 = local write "SB MaxShear"(w868) -> ()
                        }
                        frame "Permiability" {
                          n394 = Decimal String To Number(string=w875) -> (number=w874:i32)  [unwired: 2 in, 1 out]
                          n395 = Greater Than 0?(x=w874) -> (x > 0?=w873:bool)
                          n396 = local write "Perm MaxTime"(w873) -> ()
                        }
                        frame "SP" {
                          n397 = Decimal String To Number(string=w880) -> (number=w879:i32)  [unwired: 2 in, 1 out]
                          n398 = Greater Than 0?(x=w879) -> (x > 0?=w878:bool)
                          n399 = local write "SP Stop .Time"(w878) -> ()
                        }
                        frame "UCT" {
                          n400 = Decimal String To Number(string=w885) -> (number=w884:i32)  [unwired: 2 in, 1 out]
                          n401 = Greater Than 0?(x=w884) -> (x > 0?=w883:bool)
                          n402 = local write "UCT MaxDev"(w883) -> ()
                        }
                      }
                    }
                    frame 3 {
                      n403 = case shown="\"SP\"" w890 {
                        selector: w890 -> [w893 w898 w903 w907 w911 w915 w919 w923 w927 w931]
                        tunnel: [w894 w899 w904 w908 w912 w916 w920 w924 w928 w932] -> w892
                        tunnel: w891 -> [w894 w899 w904 w908 w912 w916 w920 w924 w928 w932]
                        tunnel: w888 -> [_ w897 w902 w906 w910 w914 w918 w922 w926 w930]
                        tunnel: [w893 w898 w903 w907 w911 w915 w919 w923 w927 w931] -> w889
                        frame Default {
                        }
                        frame "Consolidation" {
                          n404 = Fract/Exp String To Number(string=w897) -> (number=w896:dbl)  [unwired: 3 in, 1 out]
                          n405 = call "Main - Seconds to Time (SubVI).vi"("Seconds"=w896) -> ("Time"=w895:timestamp)  [unwired: 9 in, 1 out]
                          n406 = local write "Cons Stop Time"(w895) -> ()
                        }
                        frame "Saturation" {
                          n407 = Fract/Exp String To Number(string=w902) -> (number=w901:dbl)  [unwired: 3 in, 1 out]
                          n408 = call "Main - Seconds to Time (SubVI).vi"("Seconds"=w901) -> ("Time"=w900:timestamp)  [unwired: 9 in, 1 out]
                          n409 = local write "Sat Stop Time"(w900) -> ()
                        }
                        frame "Iso Consolidation" {
                          # "make it empty"
                          n410 = Decimal String To Number(string=w906) -> (number=w905:i32)  [unwired: 2 in, 1 out]
                          n411 = Greater Than 0?(x=w905) -> ()  [unwired: 1 out]
                        }
                        frame "TS" {
                          n412 = Fract/Exp String To Number(string=w910) -> (number=w909:dbl)  [unwired: 3 in, 1 out]
                          n413 = local write "TS MaxDev Value"(w909) -> ()
                        }
                        frame "TUU" {
                          n414 = Fract/Exp String To Number(string=w914) -> (number=w913:dbl)  [unwired: 3 in, 1 out]
                          n415 = local write "TUU MaxDev Value"(w913) -> ()
                        }
                        frame "Shearbox" {
                          n416 = Fract/Exp String To Number(string=w918) -> (number=w917:dbl)  [unwired: 3 in, 1 out]
                          n417 = local write "SB MaxShear Value"(w917) -> ()
                        }
                        frame "Permiability" {
                          n418 = Fract/Exp String To Number(string=w922) -> (number=w921:dbl)  [unwired: 3 in, 1 out]
                          n419 = local write "Perm Reset Value"(w921) -> ()
                        }
                        frame "SP" {
                          n420 = Fract/Exp String To Number(string=w926) -> (number=w925:dbl)  [unwired: 3 in, 1 out]
                          n421 = local write "SP Stop Stress"(w925) -> ()
                        }
                        frame "UCT" {
                          n422 = Fract/Exp String To Number(string=w930) -> (number=w929:dbl)  [unwired: 3 in, 1 out]
                          n423 = local write "UCT MaxDev Value"(w929) -> ()
                        }
                      }
                    }
                    frame 4 {
                      n424 = case shown="\"UCT\"" w935 {
                        selector: w935 -> [w938 w943 w947 w951 w956 w961 w966 w971 w976 w981]
                        tunnel: [w939 w944 w948 w952 w957 w962 w967 w972 w977 w982] -> w937
                        tunnel: w936 -> [w939 w944 w948 w952 w957 w962 w967 w972 w977 w982]
                        tunnel: w933 -> [_ w942 w946 w950 w955 w960 w965 w970 w975 w980]
                        tunnel: [w938 w943 w947 w951 w956 w961 w966 w971 w976 w981] -> w934
                        frame Default {
                        }
                        frame "Consolidation" {
                          n425 = Fract/Exp String To Number(string=w942) -> (number=w941:dbl)  [unwired: 3 in, 1 out]
                          n426 = call "Main - Seconds to Time (SubVI).vi"("Seconds"=w941) -> ("Time string"=w940:string)  [unwired: 9 in, 1 out]
                          n427 = local write "Cons Stop Time2"(w940) -> ()
                        }
                        frame "Saturation" {
                          n428 = Fract/Exp String To Number(string=w946) -> (number=w945:dbl)  [unwired: 3 in, 1 out]
                          n429 = local write "Sat Stop VC"(w945) -> ()
                        }
                        frame "Iso Consolidation" {
                          n430 = Fract/Exp String To Number(string=w950) -> (number=w949:dbl)  [unwired: 3 in, 1 out]
                          n431 = local write "Iso Stop PP"(w949) -> ()
                        }
                        frame "TS" {
                          n432 = Fract/Exp String To Number(string=w955) -> (number=w954:dbl)  [unwired: 3 in, 1 out]
                          n433 = Greater Than 0?(x=w954) -> (x > 0?=w953:bool)
                          n434 = local write "TS Return"(w953) -> ()
                        }
                        frame "TUU" {
                          n435 = Fract/Exp String To Number(string=w960) -> (number=w959:dbl)  [unwired: 3 in, 1 out]
                          n436 = Greater Than 0?(x=w959) -> (x > 0?=w958:bool)
                          n437 = local write "TUU Return"(w958) -> ()
                        }
                        frame "Shearbox" {
                          n438 = Fract/Exp String To Number(string=w965) -> (number=w964:dbl)  [unwired: 3 in, 1 out]
                          n439 = Greater Than 0?(x=w964) -> (x > 0?=w963:bool)
                          n440 = local write "SB Return"(w963) -> ()
                        }
                        frame "Permiability" {
                          n441 = Fract/Exp String To Number(string=w970) -> (number=w969:dbl)  [unwired: 3 in, 1 out]
                          n442 = Greater Than 0?(x=w969) -> (x > 0?=w968:bool)
                          n443 = local write "Perm Reset"(w968) -> ()
                        }
                        frame "SP" {
                          n444 = Fract/Exp String To Number(string=w975) -> (number=w974:dbl)  [unwired: 3 in, 1 out]
                          n445 = Greater Than 0?(x=w974) -> (x > 0?=w973:bool)
                          n446 = local write "SP Stop .MaxTime"(w973) -> ()
                        }
                        frame "UCT" {
                          n447 = Fract/Exp String To Number(string=w980) -> (number=w979:dbl)  [unwired: 3 in, 1 out]
                          n448 = Greater Than 0?(x=w979) -> (x > 0?=w978:bool)
                          n449 = local write "UCT Return"(w978) -> ()
                        }
                      }
                    }
                    frame 5 {
                      n450 = case shown="\"SP\"" w985 {
                        selector: w985 -> [w988 w992 w997 w1002 w1007 w1012 w1017 w1022 w1027 w1032]
                        tunnel: [w989 w993 w998 w1003 w1008 w1013 w1018 w1023 w1028 w1033] -> w987
                        tunnel: w986 -> [w989 w993 w998 w1003 w1008 w1013 w1018 w1023 w1028 w1033]
                        tunnel: w983 -> [_ w991 w996 w1001 w1006 w1011 w1016 w1021 w1026 w1031]
                        tunnel: [w988 w992 w997 w1002 w1007 w1012 w1017 w1022 w1027 w1032] -> w984
                        frame Default {
                        }
                        frame "Consolidation" {
                          n451 = Fract/Exp String To Number(string=w991) -> (number=w990:dbl)  [unwired: 3 in, 1 out]
                          n452 = local write "Cons Stop Disp 2"(w990) -> ()
                        }
                        frame "Saturation" {
                          n453 = Fract/Exp String To Number(string=w996) -> (number=w995:dbl)  [unwired: 3 in, 1 out]
                          n454 = call "Main - Seconds to Time (SubVI).vi"("Seconds"=w995) -> ("Time"=w994:timestamp)  [unwired: 9 in, 1 out]
                          n455 = local write "Sat Stop Time2"(w994) -> ()
                        }
                        frame "Iso Consolidation" {
                          n456 = Fract/Exp String To Number(string=w1001) -> (number=w1000:dbl)  [unwired: 3 in, 1 out]
                          n457 = call "Main - Seconds to Time (SubVI).vi"("Seconds"=w1000) -> ("Time string"=w999:string)  [unwired: 9 in, 1 out]
                          n458 = local write "Iso Stop Time"(w999) -> ()
                        }
                        frame "TS" {
                          n459 = Fract/Exp String To Number(string=w1006) -> (number=w1005:dbl)  [unwired: 3 in, 1 out]
                          n460 = Greater Than 0?(x=w1005) -> (x > 0?=w1004:bool)
                          n461 = local write "TS Reset"(w1004) -> ()
                        }
                        frame "TUU" {
                          n462 = Fract/Exp String To Number(string=w1011) -> (number=w1010:dbl)  [unwired: 3 in, 1 out]
                          n463 = Greater Than 0?(x=w1010) -> (x > 0?=w1009:bool)
                          n464 = local write "TUU Reset"(w1009) -> ()
                        }
                        frame "Shearbox" {
                          n465 = Fract/Exp String To Number(string=w1016) -> (number=w1015:dbl)  [unwired: 3 in, 1 out]
                          n466 = Greater Than 0?(x=w1015) -> (x > 0?=w1014:bool)
                          n467 = local write "SB Reset"(w1014) -> ()
                        }
                        frame "UCT" {
                          n468 = Fract/Exp String To Number(string=w1021) -> (number=w1020:dbl)  [unwired: 3 in, 1 out]
                          n469 = Greater Than 0?(x=w1020) -> (x > 0?=w1019:bool)
                          n470 = local write "UCT Reset"(w1019) -> ()
                        }
                        frame "Permiability" {
                          n471 = Fract/Exp String To Number(string=w1026) -> (number=w1025:dbl)  [unwired: 3 in, 1 out]
                          n472 = Greater Than 0?(x=w1025) -> (x > 0?=w1024:bool)
                          n473 = local write "Perm Ratio"(w1024) -> ()
                        }
                        frame "SP" {
                          n474 = Fract/Exp String To Number(string=w1031) -> (number=w1030:dbl)  [unwired: 3 in, 1 out]
                          n475 = call "Main - Seconds to Time (SubVI).vi"("Seconds"=w1030) -> ("Time string"=w1029:string)  [unwired: 9 in, 1 out]
                          n476 = local write "SP Stop Max Time"(w1029) -> ()
                        }
                      }
                    }
                    frame 6 {
                      n477 = case shown="\"Permiability\"" w1036 {
                        selector: w1036 -> [w1039 w1044 w1049 w1053 w1057 w1061 w1065 w1069 w1073]
                        tunnel: [w1040 w1045 w1050 w1054 w1058 w1062 w1066 w1070 w1074] -> w1038
                        tunnel: w1037 -> [w1040 w1045 w1050 w1054 w1058 w1062 w1066 w1070 w1074]
                        tunnel: w1034 -> [_ w1042 w1048 w1052 w1056 w1060 w1064 w1068 w1072]
                        tunnel: [w1039 w1044 w1049 w1053 w1057 w1061 w1065 w1069 w1073] -> w1035
                        frame Default {
                        }
                        frame "Consolidation" {
                          n478 = Decimal String To Number(string=w1042) -> (number=w1043:i32)  [unwired: 2 in, 1 out]
                          n479 = Greater Than 0?(x=w1043) -> (x > 0?=w1041:bool)
                          n480 = local write "Cons Stop Swell"(w1041) -> ()
                        }
                        frame "Saturation" {
                          n481 = Decimal String To Number(string=w1048) -> (number=w1047:i32)  [unwired: 2 in, 1 out]
                          n482 = Greater Than 0?(x=w1047) -> (x > 0?=w1046:bool)
                          n483 = local write "Sat Stop .B"(w1046) -> ()
                        }
                        frame "Iso Consolidation" {
                          n484 = Fract/Exp String To Number(string=w1052) -> (number=w1051:dbl)  [unwired: 3 in, 1 out]
                          n485 = local write "Iso Stop VC"(w1051) -> ()
                        }
                        frame "TS" {
                          n486 = Fract/Exp String To Number(string=w1056) -> (number=w1055:dbl)  [unwired: 3 in, 1 out]
                          n487 = local write "TS Reset Value"(w1055) -> ()
                        }
                        frame "TUU" {
                          n488 = Fract/Exp String To Number(string=w1060) -> (number=w1059:dbl)  [unwired: 3 in, 1 out]
                          n489 = local write "TUU Reset Value"(w1059) -> ()
                        }
                        frame "UCT" {
                          n490 = Fract/Exp String To Number(string=w1064) -> (number=w1063:dbl)  [unwired: 3 in, 1 out]
                          n491 = local write "UCT Reset Value"(w1063) -> ()
                        }
                        frame "Permiability" {
                          n492 = Fract/Exp String To Number(string=w1068) -> (number=w1067:dbl)  [unwired: 3 in, 1 out]
                          n493 = local write "Perm Ratio More"(w1067) -> ()
                        }
                        frame "Shearbox" {
                          n494 = Fract/Exp String To Number(string=w1072) -> (number=w1071:dbl)  [unwired: 3 in, 1 out]
                          n495 = local write "SB Reset Value"(w1071) -> ()
                        }
                      }
                    }
                    frame 7 {
                      n496 = case shown="\"Permiability\"" w1077 {
                        selector: w1077 -> [w1080 w1082 w1086 w1090 w1095]
                        tunnel: [w1081 w1083 w1087 w1091 w1096] -> w1079
                        tunnel: w1078 -> [w1081 w1083 w1087 w1091 w1096]
                        tunnel: w1075 -> [_ _ w1085 w1089 w1094]
                        tunnel: [w1080 w1082 w1086 w1090 w1095] -> w1076
                        frame Default {
                        }
                        frame "Consolidation" {
                        }
                        frame "Saturation" {
                          n497 = Fract/Exp String To Number(string=w1085) -> (number=w1084:dbl)  [unwired: 3 in, 1 out]
                          n498 = local write "Sat Stop B"(w1084) -> ()
                        }
                        frame "Permiability" {
                          n499 = Fract/Exp String To Number(string=w1089) -> (number=w1088:dbl)  [unwired: 3 in, 1 out]
                          n500 = local write "Perm Ratio Less"(w1088) -> ()
                        }
                        frame "Iso Consolidation" {
                          n501 = Fract/Exp String To Number(string=w1094) -> (number=w1093:dbl)  [unwired: 3 in, 1 out]
                          n502 = call "Main - Seconds to Time (SubVI).vi"("Seconds"=w1093) -> ("Time"=w1092:timestamp)  [unwired: 9 in, 1 out]
                          n503 = local write "Iso Stop Time2"(w1092) -> ()
                        }
                      }
                    }
                    frame 8 {
                      n504 = case shown="\"Permiability\"" w1099 {
                        selector: w1099 -> [w1102 w1104 w1109 w1114]
                        tunnel: [w1103 w1105 w1110 w1115] -> w1101
                        tunnel: w1100 -> [w1103 w1105 w1110 w1115]
                        tunnel: w1097 -> [_ _ w1108 w1113]
                        tunnel: [w1102 w1104 w1109 w1114] -> w1098
                        frame Default {
                        }
                        frame "Consolidation" {
                        }
                        frame "Saturation" {
                          n505 = Fract/Exp String To Number(string=w1108) -> (number=w1107:dbl)  [unwired: 3 in, 1 out]
                          n506 = call "Main - Seconds to Time (SubVI).vi"("Seconds"=w1107) -> ("Time string"=w1106:string)  [unwired: 9 in, 1 out]
                          n507 = local write "Sat Stop Time3"(w1106) -> ()
                        }
                        frame "Permiability" {
                          n508 = Fract/Exp String To Number(string=w1113) -> (number=w1112:dbl)  [unwired: 3 in, 1 out]
                          n509 = call "Main - Seconds to Time (SubVI).vi"("Seconds"=w1112) -> ("Time string"=w1111:string)  [unwired: 9 in, 1 out]
                          n510 = local write "Perm Ratio Time"(w1111) -> ()
                        }
                      }
                    }
                  }
                }
              }
              frame True {
              }
            }
          }
          frame "Save" {
            n511 = property on="Test Type" class="Ring (strict)"(error in=w1126) -> (error out=w1127:errorcluster, "RingText.Text"=w1124:string)  [unwired: 1 in, 1 out]
            n512 = local read "Start Enable"() -> (w1119:bool)
            n513 = local read "Stop Enable"() -> (w1118:bool)
            n514 = for {
              tunnel: w1123 -> [w1141]
              shift-right: [w1142] -> w1122
              shift-left: w1127 -> [w1140]
              tunnel: string[] ["Start Condition", "Log Condition", "Stop Condition"] ("TestPlan Name") -> [w1139] mode=indexing
              tunnel: w1124 -> [w1136]
              tunnel: w1119 -> [w1134]
              tunnel: w1118 -> [w1133]
              i -> [w1137]
              n515 = case shown="2" w1137 {
                tunnel: [string[] ["Test Type", "Data 1", "Data 2", "Data 3", "Data 4", "Data 5", "Data 6", "Data 7", "Data 8"] ("Value") string[] ["Test Type", "Data 1", "Data 2", "Data 3", "Data 4", "Data 5"] ("Value") string[] ["Test Type", "Data 1", "Data 2", "Data 3", "Data 4", "Data 5", "Data 6", "Data 7", "Data 8"] ("Value")] -> w1138
                tunnel: w1136 -> [w1146 w1285 w1446]
                tunnel: [w1145 w1284 w1445] -> w1135
                tunnel: w1134 -> [w1144 _ _]
                tunnel: w1133 -> [_ _ w1444]
                frame 0, Default {
                  n516 = case shown="True" w1144 {
                    tunnel: w1146 -> [w1148 w1153]
                    tunnel: [w1149 w1152] -> w1145
                    frame False {
                      n517 = Build Array(w1148, "Disabled") -> (w1149:string[])
                    }
                    frame True {
                      n518 = local read "Start Tab"() -> (w1151:T3)
                      n519 = case shown="\"Saturation\"" w1151 {
                        selector: w1151 -> [_ w1158 w1175 w1183 w1191 w1216 w1237 w1250 w1260 w1264 _]
                        tunnel: w1153 -> [w1156 w1168 w1179 w1186 w1190 w1215 w1236 w1249 w1259 w1266 w1273]
                        tunnel: [w1155 w1167 w1178 w1185 w1199 w1220 w1241 w1254 w1261 w1265 w1272] -> w1152
                        frame "User Defined" {
                          w1154 = "" ("element")
                          n520 = Build Array(w1156, w1154, w1154, w1154) -> (w1155:string[])
                        }
                        frame "Consolidation" {
                          n521 = call "Main - Time to Seconds (SubVI).vi"("Time"="Cons Start Delay") -> ("Seconds"=w1162:dbl)  [unwired: 10 in]
                          n522 = Boolean To (0,1)(Boolean="Cons Start .Delay") -> (0, 1=w1163:i16)
                          n523 = Number To Fractional String(number=w1158) -> (F-format string=w1157:string)  [unwired: 3 in]
                          n524 = Number To Fractional String(number="Cons Start VS") -> (F-format string=w1161:string)  [unwired: 3 in]
                          n525 = Number To Decimal String(number=w1163) -> (decimal integer string=w1160:string)  [unwired: 1 in]
                          n526 = Number To Fractional String(number=w1162) -> (F-format string=w1159:string)  [unwired: 3 in]
                          n527 = Build Array(w1168, w1157, w1161, w1160, w1159) -> (w1167:string[])
                        }
                        frame "Saturation" {
                          n528 = Boolean To (0,1)(Boolean="Sat Start BP") -> (0, 1=w1171:i16)
                          n529 = Number To Fractional String(number=w1175) -> (F-format string=w1174:string)  [unwired: 3 in]
                          n530 = Number To Fractional String(number="Sat CP") -> (F-format string=w1177:string)  [unwired: 3 in]
                          n531 = Number To Fractional String(number="Sat BP") -> (F-format string=w1176:string)  [unwired: 3 in]
                          n532 = Number To Decimal String(number=w1171) -> (decimal integer string=w1169:string)  [unwired: 1 in]
                          n533 = Build Array(w1179, w1174, w1177, w1176, w1169) -> (w1178:string[])
                        }
                        frame "Iso Consolidation" {
                          w1180 = "" ("element")
                          n534 = Number To Fractional String(number=w1183) -> (F-format string=w1182:string)  [unwired: 3 in]
                          n535 = Number To Fractional String(number="Iso BP") -> (F-format string=w1184:string)  [unwired: 3 in]
                          n536 = Build Array(w1186, w1182, w1184, w1180, w1180) -> (w1185:string[])
                        }
                        frame "TS" {
                          n537 = Boolean To (0,1)(Boolean="TS Engage") -> (0, 1=w1196:i16)
                          n538 = Number To Fractional String(number=w1191) -> (F-format string=w1189:string)  [unwired: 3 in]
                          n539 = Number To Fractional String(number="TS Shear Speed") -> (F-format string=w1200:string)  [unwired: 3 in]
                          n540 = Number To Decimal String(number=w1196) -> (decimal integer string=w1201:string)  [unwired: 1 in]
                          n541 = Number To Fractional String(number="TS Engage Speed") -> (F-format string=w1194:string)  [unwired: 3 in]
                          n542 = Number To Fractional String(number="TS Load Change") -> (F-format string=w1192:string)  [unwired: 3 in]
                          n543 = Number To Decimal String(number="TS Drain") -> (decimal integer string=w1187:string)  [unwired: 1 in]
                          n544 = Build Array(w1190, w1189, w1200, w1201, w1194, w1192, w1187) -> (w1199:string[])
                        }
                        frame "TUU" {
                          n545 = call "Main - Time to Seconds (SubVI).vi"("Time"="TUU Start Delay") -> ("Seconds"=w1203:dbl)  [unwired: 10 in]
                          n546 = Boolean To (0,1)(Boolean="TUU Engage") -> (0, 1=w1219:i16)
                          n547 = Boolean To (0,1)(Boolean="TUU Start .Delay") -> (0, 1=w1207:i16)
                          n548 = Number To Fractional String(number=w1216) -> (F-format string=w1214:string)  [unwired: 3 in]
                          n549 = Number To Fractional String(number="TUU Shear Speed") -> (F-format string=w1221:string)  [unwired: 3 in]
                          n550 = Number To Decimal String(number=w1219) -> (decimal integer string=w1222:string)  [unwired: 1 in]
                          n551 = Number To Fractional String(number="TUU Engage Speed") -> (F-format string=w1218:string)  [unwired: 3 in]
                          n552 = Number To Fractional String(number="TUU Load Change") -> (F-format string=w1217:string)  [unwired: 3 in]
                          n553 = Number To Fractional String(number="TUU Confining Pressure") -> (F-format string=w1208:string)  [unwired: 3 in]
                          n554 = Number To Decimal String(number=w1207) -> (decimal integer string=w1206:string)  [unwired: 1 in]
                          n555 = Number To Fractional String(number=w1203) -> (F-format string=w1205:string)  [unwired: 3 in]
                          n556 = Build Array(w1215, w1214, w1221, w1222, w1218, w1217, w1208, w1206, w1205) -> (w1220:string[])
                        }
                        frame "Shearbox" {
                          n557 = call "Main - Time to Seconds (SubVI).vi"("Time"="SB Start Delay") -> ("Seconds"=w1230:dbl)  [unwired: 10 in]
                          n558 = Boolean To (0,1)(Boolean="SB Engage") -> (0, 1=w1240:i16)
                          n559 = Boolean To (0,1)(Boolean="SB Start .Delay") -> (0, 1=w1233:i16)
                          n560 = Number To Fractional String(number=w1237) -> (F-format string=w1235:string)  [unwired: 3 in]
                          n561 = Number To Fractional String(number="SB Shear Speed") -> (F-format string=w1242:string)  [unwired: 3 in]
                          n562 = Number To Decimal String(number=w1240) -> (decimal integer string=w1243:string)  [unwired: 1 in]
                          n563 = Number To Fractional String(number="SB Engage Speed") -> (F-format string=w1239:string)  [unwired: 3 in]
                          n564 = Number To Fractional String(number="SB Load Change") -> (F-format string=w1238:string)  [unwired: 3 in]
                          n565 = Number To Fractional String(number="SB Vertical Load") -> (F-format string=w1234:string)  [unwired: 3 in]
                          n566 = Number To Decimal String(number=w1233) -> (decimal integer string=w1232:string)  [unwired: 1 in]
                          n567 = Number To Fractional String(number=w1230) -> (F-format string=w1231:string)  [unwired: 3 in]
                          n568 = Build Array(w1236, w1235, w1242, w1243, w1239, w1238, w1234, w1232, w1231) -> (w1241:string[])
                        }
                        frame "UCT" {
                          n569 = Boolean To (0,1)(Boolean="UCT Engage") -> (0, 1=w1253:i16)
                          n570 = Number To Fractional String(number=w1250) -> (F-format string=w1248:string)  [unwired: 3 in]
                          n571 = Number To Fractional String(number="UCT Shear Speed") -> (F-format string=w1255:string)  [unwired: 3 in]
                          n572 = Number To Decimal String(number=w1253) -> (decimal integer string=w1256:string)  [unwired: 1 in]
                          n573 = Number To Fractional String(number="UCT Engage Speed") -> (F-format string=w1252:string)  [unwired: 3 in]
                          n574 = Number To Fractional String(number="UCT Load Change") -> (F-format string=w1251:string)  [unwired: 3 in]
                          n575 = Build Array(w1249, w1248, w1255, w1256, w1252, w1251) -> (w1254:string[])
                        }
                        frame "Permiability" {
                          n576 = Number To Fractional String(number=w1260) -> (F-format string=w1258:string)  [unwired: 3 in]
                          n577 = Number To Fractional String(number="Perm DP") -> (F-format string=w1262:string)  [unwired: 3 in]
                          n578 = Build Array(w1259, w1258, w1262) -> (w1261:string[])
                        }
                        frame "SP" {
                          n579 = Number To Fractional String(number=w1264) -> (F-format string=w1263:string)  [unwired: 3 in]
                          n580 = Build Array(w1266, w1263) -> (w1265:string[])
                        }
                        frame "Others", Default {
                          n581 = local read "Sub Start"() -> (w1267:enum32{"1", "2"})
                          n582 = Number To Decimal String(number=w1267) -> (decimal integer string=w1279:string)  [unwired: 1 in]
                          n583 = Number To Decimal String(number="Start Delay") -> (decimal integer string=w1280:string)  [unwired: 1 in]
                          n584 = Number To Fractional String(number="Start load", precision (6)=i16 4) -> (F-format string=w1271:string)  [unwired: 2 in]
                          n585 = Index Array(array="Start Load", index (col)=1 ("disabled index (col)")) -> (element=w1270:string[])  [unwired: 1 in]
                          n586 = Build Array (concatenate)(w1271, w1270) -> (w1269:string[])
                          n587 = Array To Spreadsheet String(delimiter (Tab)=",", array=w1269, 3:"" ("format string")) -> (spreadsheet string=w1282:string)
                          n588 = Build Array(w1273, w1279, w1280, w1282) -> (w1272:string[])
                        }
                      }
                    }
                  }
                }
                frame 1 {
                  n589 = local read "Log Tab"() -> (w1283:T4)
                  n590 = case shown="\"Saturation\"" w1283 {
                    tunnel: w1285 -> [w1303 w1322 w1341 w1362 w1383 w1402 w1423 w1432 w1439 w1440 w1442]
                    tunnel: [w1297 w1316 w1335 w1356 w1377 w1396 w1417 w1430 w1437 w1441 w1443] -> w1284
                    frame "Consolidation" {
                      n591 = local read "Cons Log Select"() -> (w1291:enum32{"1", "2"})
                      n592 = call "Main - Time to Seconds (SubVI).vi"("Time"="Cons Log Delay") -> ("Seconds"=w1287:dbl)  [unwired: 10 in]
                      n593 = Number To Decimal String(number=w1291) -> (decimal integer string=w1302:string)  [unwired: 1 in]
                      n594 = Number To Fractional String(number=w1287) -> (F-format string=w1296:string)  [unwired: 3 in]
                      n595 = Index Array(array="Cons LogTime", index (col)=1 ("disabled index (col)")) -> (element=w1301:string[])  [unwired: 1 in]
                      n596 = Index Array(array="Cons LogDisp", index (col)=1 ("disabled index (col)")) -> (element=w1300:string[])  [unwired: 1 in]
                      n597 = Array To Spreadsheet String(delimiter (Tab)=",", array=w1301, 3:"" ("format string")) -> (spreadsheet string=w1295:string)
                      n598 = Array To Spreadsheet String(delimiter (Tab)=",", array=w1300, 3:"" ("format string")) -> (spreadsheet string=w1294:string)
                      n599 = Build Array(w1303, w1302, w1296, w1295, w1294) -> (w1297:string[])
                    }
                    frame "Saturation" {
                      n600 = local read "Sat Log Select"() -> (w1309:enum32{"1", "2"})
                      n601 = call "Main - Time to Seconds (SubVI).vi"("Time"="Sat Log Delay") -> ("Seconds"=w1310:dbl)  [unwired: 10 in]
                      n602 = Number To Decimal String(number=w1309) -> (decimal integer string=w1321:string)  [unwired: 1 in]
                      n603 = Number To Fractional String(number=w1310) -> (F-format string=w1315:string)  [unwired: 3 in]
                      n604 = Index Array(array="Sat LogTime", index (col)=1 ("disabled index (col)")) -> (element=w1320:string[])  [unwired: 1 in]
                      n605 = Index Array(array="Sat LogDisp", index (col)=1 ("disabled index (col)")) -> (element=w1319:string[])  [unwired: 1 in]
                      n606 = Array To Spreadsheet String(delimiter (Tab)=",", array=w1320, 3:"" ("format string")) -> (spreadsheet string=w1314:string)
                      n607 = Array To Spreadsheet String(delimiter (Tab)=",", array=w1319, 3:"" ("format string")) -> (spreadsheet string=w1313:string)
                      n608 = Build Array(w1322, w1321, w1315, w1314, w1313) -> (w1316:string[])
                    }
                    frame "Iso Consolidation" {
                      n609 = local read "Iso Log Select"() -> (w1328:enum32{"1", "2"})
                      n610 = call "Main - Time to Seconds (SubVI).vi"("Time"="Iso Log Delay") -> ("Seconds"=w1329:dbl)  [unwired: 10 in]
                      n611 = Number To Decimal String(number=w1328) -> (decimal integer string=w1340:string)  [unwired: 1 in]
                      n612 = Number To Fractional String(number=w1329) -> (F-format string=w1334:string)  [unwired: 3 in]
                      n613 = Index Array(array="Iso LogTime", index (col)=1 ("disabled index (col)")) -> (element=w1339:string[])  [unwired: 1 in]
                      n614 = Index Array(array="Iso LogDisp", index (col)=1 ("disabled index (col)")) -> (element=w1338:string[])  [unwired: 1 in]
                      n615 = Array To Spreadsheet String(delimiter (Tab)=",", array=w1339, 3:"" ("format string")) -> (spreadsheet string=w1333:string)
                      n616 = Array To Spreadsheet String(delimiter (Tab)=",", array=w1338, 3:"" ("format string")) -> (spreadsheet string=w1332:string)
                      n617 = Build Array(w1341, w1340, w1334, w1333, w1332) -> (w1335:string[])
                    }
                    frame "TS" {
                      n618 = local read "TS Log Select"() -> (w1344:enum32{"1", "3", "2"})
                      n619 = call "Main - Time to Seconds (SubVI).vi"("Time"="TS Log Delay") -> ("Seconds"=w1350:dbl)  [unwired: 10 in]
                      n620 = Number To Decimal String(number=w1344) -> (decimal integer string=w1361:string)  [unwired: 1 in]
                      n621 = Number To Fractional String(number=w1350) -> (F-format string=w1355:string)  [unwired: 3 in]
                      n622 = Index Array(array="TS LogTime", index (col)=1 ("disabled index (col)")) -> (element=w1360:string[])  [unwired: 1 in]
                      n623 = Index Array(array="TS LogDisp", index (col)=1 ("disabled index (col)")) -> (element=w1359:string[])  [unwired: 1 in]
                      n624 = Number To Fractional String(number="TS LogAxial") -> (F-format string=w1345:string)  [unwired: 3 in]
                      n625 = Array To Spreadsheet String(delimiter (Tab)=",", array=w1360, 3:"" ("format string")) -> (spreadsheet string=w1354:string)
                      n626 = Array To Spreadsheet String(delimiter (Tab)=",", array=w1359, 3:"" ("format string")) -> (spreadsheet string=w1353:string)
                      n627 = Build Array(w1362, w1361, w1355, w1354, w1353, w1345) -> (w1356:string[])
                    }
                    frame "TUU" {
                      n628 = local read "TUU Log Select"() -> (w1369:enum32{"1", "3", "2"})
                      n629 = call "Main - Time to Seconds (SubVI).vi"("Time"="TUU Log Delay") -> ("Seconds"=w1371:dbl)  [unwired: 10 in]
                      n630 = Number To Decimal String(number=w1369) -> (decimal integer string=w1382:string)  [unwired: 1 in]
                      n631 = Number To Fractional String(number=w1371) -> (F-format string=w1376:string)  [unwired: 3 in]
                      n632 = Index Array(array="TUU LogTime", index (col)=1 ("disabled index (col)")) -> (element=w1381:string[])  [unwired: 1 in]
                      n633 = Index Array(array="TUU LogDisp", index (col)=1 ("disabled index (col)")) -> (element=w1380:string[])  [unwired: 1 in]
                      n634 = Number To Fractional String(number="TUU LogAxial") -> (F-format string=w1370:string)  [unwired: 3 in]
                      n635 = Array To Spreadsheet String(delimiter (Tab)=",", array=w1381, 3:"" ("format string")) -> (spreadsheet string=w1375:string)
                      n636 = Array To Spreadsheet String(delimiter (Tab)=",", array=w1380, 3:"" ("format string")) -> (spreadsheet string=w1374:string)
                      n637 = Build Array(w1383, w1382, w1376, w1375, w1374, w1370) -> (w1377:string[])
                    }
                    frame "Shearbox" {
                      n638 = local read "SB Log Select"() -> (w1389:enum32{"1", "2"})
                      n639 = call "Main - Time to Seconds (SubVI).vi"("Time"="SB Log Delay") -> ("Seconds"=w1390:dbl)  [unwired: 10 in]
                      n640 = Number To Decimal String(number=w1389) -> (decimal integer string=w1401:string)  [unwired: 1 in]
                      n641 = Number To Fractional String(number=w1390) -> (F-format string=w1395:string)  [unwired: 3 in]
                      n642 = Index Array(array="SB LogTime", index (col)=1 ("disabled index (col)")) -> (element=w1400:string[])  [unwired: 1 in]
                      n643 = Index Array(array="SB LogDisp", index (col)=1 ("disabled index (col)")) -> (element=w1399:string[])  [unwired: 1 in]
                      n644 = Array To Spreadsheet String(delimiter (Tab)=",", array=w1400, 3:"" ("format string")) -> (spreadsheet string=w1394:string)
                      n645 = Array To Spreadsheet String(delimiter (Tab)=",", array=w1399, 3:"" ("format string")) -> (spreadsheet string=w1393:string)
                      n646 = Build Array(w1402, w1401, w1395, w1394, w1393) -> (w1396:string[])
                    }
                    frame "UCT" {
                      n647 = local read "UCT Log Select"() -> (w1409:enum32{"1", "3", "2"})
                      n648 = call "Main - Time to Seconds (SubVI).vi"("Time"="UCT Log Delay") -> ("Seconds"=w1411:dbl)  [unwired: 10 in]
                      n649 = Number To Decimal String(number=w1409) -> (decimal integer string=w1422:string)  [unwired: 1 in]
                      n650 = Number To Fractional String(number=w1411) -> (F-format string=w1416:string)  [unwired: 3 in]
                      n651 = Index Array(array="UCT LogTime", index (col)=1 ("disabled index (col)")) -> (element=w1421:string[])  [unwired: 1 in]
                      n652 = Index Array(array="UCT LogDisp", index (col)=1 ("disabled index (col)")) -> (element=w1420:string[])  [unwired: 1 in]
                      n653 = Number To Fractional String(number="UCT LogAxial") -> (F-format string=w1410:string)  [unwired: 3 in]
                      n654 = Array To Spreadsheet String(delimiter (Tab)=",", array=w1421, 3:"" ("format string")) -> (spreadsheet string=w1415:string)
                      n655 = Array To Spreadsheet String(delimiter (Tab)=",", array=w1420, 3:"" ("format string")) -> (spreadsheet string=w1414:string)
                      n656 = Build Array(w1423, w1422, w1416, w1415, w1414, w1410) -> (w1417:string[])
                    }
                    frame "Permiability" {
                      n657 = local read "Perm Log Select"() -> (w1427:enum32{"1"})
                      n658 = call "Main - Time to Seconds (SubVI).vi"("Time"="Perm Log Delay") -> ("Seconds"=w1428:dbl)  [unwired: 10 in]
                      n659 = Number To Decimal String(number=w1427) -> (decimal integer string=w1431:string)  [unwired: 1 in]
                      n660 = Number To Fractional String(number=w1428) -> (F-format string=w1429:string)  [unwired: 3 in]
                      n661 = Build Array(w1432, w1431, w1429) -> (w1430:string[])
                    }
                    frame "SP" {
                      n662 = local read "SP Log Select"() -> (w1434:enum32{"1"})
                      n663 = call "Main - Time to Seconds (SubVI).vi"("Time"="SP Log Delay") -> ("Seconds"=w1435:dbl)  [unwired: 10 in]
                      n664 = Number To Decimal String(number=w1434) -> (decimal integer string=w1438:string)  [unwired: 1 in]
                      n665 = Number To Fractional String(number=w1435) -> (F-format string=w1436:string)  [unwired: 3 in]
                      n666 = Build Array(w1439, w1438, w1436) -> (w1437:string[])
                    }
                    frame "Others", Default {
                      n667 = Build Array(w1440, w1440, w1440, w1440, w1440) -> (w1441:string[])
                    }
                    frame "User Defined" {
                      n668 = Build Array(w1442, w1442, w1442, w1442, w1442) -> (w1443:string[])
                    }
                  }
                }
                frame 2 {
                  n669 = case shown="True" w1444 {
                    tunnel: w1446 -> [_ w1452]
                    tunnel: [w1448 w1451] -> w1445
                    frame False {
                      n670 = Build Array("Disabled") -> (w1448:string[])
                    }
                    frame True {
                      n671 = local read "Stop Tab"() -> (w1450:T5)
                      n672 = case shown="\"UCT\"" w1450 {
                        tunnel: w1452 -> [w1455 w1474 w1497 w1518 w1534 w1553 w1570 w1587 w1612 w1630 w1647]
                        tunnel: [w1454 w1473 w1496 w1517 w1521 w1549 w1566 w1583 w1608 w1627 w1643] -> w1451
                        frame "User Defined" {
                          w1453 = "" ("element")
                          n673 = Build Array(w1455, w1453, w1453, w1453, w1453) -> (w1454:string[])
                        }
                        frame "Consolidation" {
                          n674 = call "Main - Time to Seconds (SubVI).vi"("Time"="Cons Stop Time") -> ("Seconds"=w1467:dbl)  [unwired: 10 in]
                          n675 = call "Main - Time to Seconds (SubVI).vi"("String?"=TRUE, "Time String"="Cons Stop Time2") -> ("Seconds"=w1468:dbl)  [unwired: 9 in]
                          n676 = Boolean To (0,1)(Boolean="Cons Stop Swell") -> (0, 1=w1460:i16)
                          n677 = Number To Decimal String(number="Cons Stop Select") -> (decimal integer string=w1471:string)  [unwired: 1 in]
                          n678 = Number To Fractional String(number="Cons Stop Disp") -> (F-format string=w1465:string)  [unwired: 3 in]
                          n679 = Number To Fractional String(number=w1467) -> (F-format string=w1464:string)  [unwired: 3 in]
                          n680 = Number To Fractional String(number=w1468) -> (F-format string=w1463:string)  [unwired: 3 in]
                          n681 = Number To Fractional String(number="Cons Stop Disp 2") -> (F-format string=w1462:string)  [unwired: 3 in]
                          n682 = Number To Decimal String(number=w1460) -> (decimal integer string=w1458:string)  [unwired: 1 in]
                          n683 = Build Array(w1474, w1471, w1465, w1464, w1463, w1462, w1458, "" ("element")) -> (w1473:string[])
                        }
                        frame "Saturation" {
                          n684 = call "Main - Time to Seconds (SubVI).vi"("String?"=TRUE, "Time String"="Sat Stop Time3") -> ("Seconds"=w1476:dbl)  [unwired: 9 in]
                          n685 = Boolean To (0,1)(Boolean="Sat Stop .B") -> (0, 1=w1479:i16)
                          n686 = call "Main - Time to Seconds (SubVI).vi"("Time"="Sat Stop Time") -> ("Seconds"=w1494:dbl)  [unwired: 10 in]
                          n687 = call "Main - Time to Seconds (SubVI).vi"("Time"="Sat Stop Time2") -> ("Seconds"=w1484:dbl)  [unwired: 10 in]
                          n688 = Number To Decimal String(number="Sat Stop Select") -> (decimal integer string=w1495:string)  [unwired: 1 in]
                          n689 = Number To Fractional String(number="Sat Stop PP") -> (F-format string=w1493:string)  [unwired: 3 in]
                          n690 = Number To Fractional String(number=w1494) -> (F-format string=w1492:string)  [unwired: 3 in]
                          n691 = Number To Fractional String(number="Sat Stop VC") -> (F-format string=w1491:string)  [unwired: 3 in]
                          n692 = Number To Fractional String(number=w1484) -> (F-format string=w1490:string)  [unwired: 3 in]
                          n693 = Number To Decimal String(number=w1479) -> (decimal integer string=w1483:string)  [unwired: 1 in]
                          n694 = Number To Fractional String(number="Sat Stop B") -> (F-format string=w1482:string)  [unwired: 3 in]
                          n695 = Number To Fractional String(number=w1476) -> (F-format string=w1475:string)  [unwired: 3 in]
                          n696 = Build Array(w1497, w1495, w1493, w1492, w1491, w1490, w1483, w1482, w1475) -> (w1496:string[])
                        }
                        frame "Iso Consolidation" {
                          n697 = Boolean To (0,1)(Boolean="Iso Stop .PP") -> (0, 1=w1507:i16)
                          n698 = Boolean To (0,1)(Boolean=FALSE) -> (0, 1=w1506:i16)
                          n699 = call "Main - Time to Seconds (SubVI).vi"("Time"="Iso Stop Time2") -> ("Seconds"=w1502:dbl)  [unwired: 10 in]
                          n700 = call "Main - Time to Seconds (SubVI).vi"("String?"=TRUE, "Time String"="Iso Stop Time") -> ("Seconds"=w1511:dbl)  [unwired: 9 in]
                          n701 = Number To Decimal String(number=w1507) -> (decimal integer string=w1516:string)  [unwired: 1 in]
                          n702 = Number To Decimal String(number="Iso Stop Select") -> (decimal integer string=w1515:string)  [unwired: 1 in]
                          n703 = Number To Decimal String(number=w1506) -> (decimal integer string=w1514:string)  [unwired: 1 in]
                          n704 = Number To Fractional String(number="Iso Stop PP") -> (F-format string=w1513:string)  [unwired: 3 in]
                          n705 = Number To Fractional String(number=w1511) -> (F-format string=w1512:string)  [unwired: 3 in]
                          n706 = Number To Fractional String(number="Iso Stop VC") -> (F-format string=w1510:string)  [unwired: 3 in]
                          n707 = Number To Fractional String(number=w1502) -> (F-format string=w1509:string)  [unwired: 3 in]
                          n708 = Build Array(w1518, w1516, w1515, w1514, w1513, w1512, w1510, w1509) -> (w1517:string[])
                        }
                        frame "Others", Default {
                          n709 = local read "Sub Stop"() -> (w1519:enum32{"1", "2"})
                          n710 = To Double Precision Float(number="Stop Time") -> (double precision float=w1527:dbl)
                          n711 = Boolean To (0,1)(Boolean="Return") -> (0, 1=w1522:i16)
                          n712 = Number To Decimal String(number=w1519) -> (decimal integer string=w1533:string)  [unwired: 1 in]
                          n713 = Number To Decimal String(number="Stop Duration") -> (decimal integer string=w1532:string)  [unwired: 1 in]
                          n714 = Number To Fractional String(number="stop load", precision (6)=i16 4) -> (F-format string=w1530:string)  [unwired: 2 in]
                          n715 = Number To Fractional String(number=w1527, precision (6)=i16 4) -> (F-format string=w1526:string)  [unwired: 2 in]
                          n716 = Number To Decimal String(number=w1522) -> (decimal integer string=w1520:string)  [unwired: 1 in]
                          n717 = Concatenate Strings(w1530, "," ("string"), w1526) -> (w1525:string)
                          n718 = Build Array(w1534, w1533, w1532, w1525, w1520) -> (w1521:string[])
                        }
                        frame "TS" {
                          n719 = Boolean To (0,1)(Boolean="TS MaxDev") -> (0, 1=w1546:i16)
                          n720 = Boolean To (0,1)(Boolean="TS Return") -> (0, 1=w1541:i16)
                          n721 = Boolean To (0,1)(Boolean="TS Reset") -> (0, 1=w1550:i16)
                          n722 = Number To Fractional String(number="TS Axial Value") -> (F-format string=w1552:string)  [unwired: 3 in]
                          n723 = Number To Decimal String(number=w1546) -> (decimal integer string=w1551:string)  [unwired: 1 in]
                          n724 = Number To Fractional String(number="TS MaxDev Value") -> (F-format string=w1544:string)  [unwired: 3 in]
                          n725 = Number To Decimal String(number=w1541) -> (decimal integer string=w1539:string)  [unwired: 1 in]
                          n726 = Number To Decimal String(number=w1550) -> (decimal integer string=w1540:string)  [unwired: 1 in]
                          n727 = Number To Fractional String(number="TS Reset Value") -> (F-format string=w1537:string)  [unwired: 3 in]
                          n728 = Build Array(w1553, w1552, w1551, w1544, w1539, w1540, w1537) -> (w1549:string[])
                        }
                        frame "TUU" {
                          n729 = Boolean To (0,1)(Boolean="TUU MaxDev") -> (0, 1=w1565:i16)
                          n730 = Boolean To (0,1)(Boolean="TUU Return") -> (0, 1=w1563:i16)
                          n731 = Boolean To (0,1)(Boolean="TUU Reset") -> (0, 1=w1567:i16)
                          n732 = Number To Fractional String(number="TUU Axial Value") -> (F-format string=w1569:string)  [unwired: 3 in]
                          n733 = Number To Decimal String(number=w1565) -> (decimal integer string=w1568:string)  [unwired: 1 in]
                          n734 = Number To Fractional String(number="TUU MaxDev Value") -> (F-format string=w1564:string)  [unwired: 3 in]
                          n735 = Number To Decimal String(number=w1563) -> (decimal integer string=w1556:string)  [unwired: 1 in]
                          n736 = Number To Decimal String(number=w1567) -> (decimal integer string=w1555:string)  [unwired: 1 in]
                          n737 = Number To Fractional String(number="TUU Reset Value") -> (F-format string=w1554:string)  [unwired: 3 in]
                          n738 = Build Array(w1570, w1569, w1568, w1564, w1556, w1555, w1554) -> (w1566:string[])
                        }
                        frame "Shearbox" {
                          n739 = Boolean To (0,1)(Boolean="SB MaxShear") -> (0, 1=w1582:i16)
                          n740 = Boolean To (0,1)(Boolean="SB Return") -> (0, 1=w1580:i16)
                          n741 = Boolean To (0,1)(Boolean="SB Reset") -> (0, 1=w1584:i16)
                          n742 = Number To Fractional String(number="SB Shear Value") -> (F-format string=w1586:string)  [unwired: 3 in]
                          n743 = Number To Decimal String(number=w1582) -> (decimal integer string=w1585:string)  [unwired: 1 in]
                          n744 = Number To Fractional String(number="SB MaxShear Value") -> (F-format string=w1581:string)  [unwired: 3 in]
                          n745 = Number To Decimal String(number=w1580) -> (decimal integer string=w1579:string)  [unwired: 1 in]
                          n746 = Number To Decimal String(number=w1584) -> (decimal integer string=w1578:string)  [unwired: 1 in]
                          n747 = Number To Fractional String(number="SB Reset Value") -> (F-format string=w1577:string)  [unwired: 3 in]
                          n748 = Build Array(w1587, w1586, w1585, w1581, w1579, w1578, w1577) -> (w1583:string[])
                        }
                        frame "Permiability" {
                          n749 = call "Main - Time to Seconds (SubVI).vi"("String?"=TRUE, "Time String"="Perm Stop Time") -> ("Seconds"=w1599:dbl)  [unwired: 9 in]
                          n750 = Boolean To (0,1)(Boolean="Perm MaxTime") -> (0, 1=w1607:i16)
                          n751 = Boolean To (0,1)(Boolean="Perm Reset") -> (0, 1=w1605:i16)
                          n752 = Boolean To (0,1)(Boolean="Perm Ratio") -> (0, 1=w1609:i16)
                          n753 = call "Main - Time to Seconds (SubVI).vi"("String?"=TRUE, "Time String"="Perm Ratio Time") -> ("Seconds"=w1590:dbl)  [unwired: 9 in]
                          n754 = Number To Fractional String(number=w1599) -> (F-format string=w1611:string)  [unwired: 3 in]
                          n755 = Number To Decimal String(number=w1607) -> (decimal integer string=w1610:string)  [unwired: 1 in]
                          n756 = Number To Fractional String(number="Perm Reset Value") -> (F-format string=w1606:string)  [unwired: 3 in]
                          n757 = Number To Decimal String(number=w1605) -> (decimal integer string=w1604:string)  [unwired: 1 in]
                          n758 = Number To Decimal String(number=w1609) -> (decimal integer string=w1603:string)  [unwired: 1 in]
                          n759 = Number To Fractional String(number="Perm Ratio More") -> (F-format string=w1602:string)  [unwired: 3 in]
                          n760 = Number To Fractional String(number="Perm Ratio Less") -> (F-format string=w1589:string)  [unwired: 3 in]
                          n761 = Number To Fractional String(number=w1590, precision (6)=w1590) -> (F-format string=w1588:string)  [unwired: 2 in]
                          n762 = Build Array(w1612, w1611, w1610, w1606, w1604, w1603, w1602, w1589, w1588) -> (w1608:string[])
                        }
                        frame "SP" {
                          n763 = call "Main - Time to Seconds (SubVI).vi"("String?"=TRUE, "Time String"="SP Stop Time") -> ("Seconds"=w1621:dbl)  [unwired: 9 in]
                          n764 = Boolean To (0,1)(Boolean="SP Stop .Time") -> (0, 1=w1626:i16)
                          n765 = Boolean To (0,1)(Boolean="SP Stop .MaxTime") -> (0, 1=w1624:i16)
                          n766 = call "Main - Time to Seconds (SubVI).vi"("String?"=TRUE, "Time String"="SP Stop Max Time") -> ("Seconds"=w1619:dbl)  [unwired: 9 in]
                          n767 = Number To Fractional String(number=w1621) -> (F-format string=w1629:string)  [unwired: 3 in]
                          n768 = Number To Decimal String(number=w1626) -> (decimal integer string=w1628:string)  [unwired: 1 in]
                          n769 = Number To Fractional String(number="SP Stop Stress") -> (F-format string=w1625:string)  [unwired: 3 in]
                          n770 = Number To Decimal String(number=w1624) -> (decimal integer string=w1623:string)  [unwired: 1 in]
                          n771 = Number To Fractional String(number=w1619, precision (6)=w1619) -> (F-format string=w1614:string)  [unwired: 2 in]
                          n772 = Build Array(w1630, w1629, w1628, w1625, w1623, w1614) -> (w1627:string[])
                        }
                        frame "UCT" {
                          n773 = Boolean To (0,1)(Boolean="UCT MaxDev") -> (0, 1=w1641:i16)
                          n774 = Boolean To (0,1)(Boolean="UCT Return") -> (0, 1=w1639:i16)
                          n775 = Boolean To (0,1)(Boolean="UCT Reset") -> (0, 1=w1644:i16)
                          n776 = Number To Fractional String(number="UCT Axial Value") -> (F-format string=w1646:string)  [unwired: 3 in]
                          n777 = Number To Decimal String(number=w1641) -> (decimal integer string=w1645:string)  [unwired: 1 in]
                          n778 = Number To Fractional String(number="UCT MaxDev Value") -> (F-format string=w1640:string)  [unwired: 3 in]
                          n779 = Number To Decimal String(number=w1639) -> (decimal integer string=w1631:string)  [unwired: 1 in]
                          n780 = Number To Decimal String(number=w1644) -> (decimal integer string=w1642:string)  [unwired: 1 in]
                          n781 = Number To Fractional String(number="UCT Reset Value") -> (F-format string=w1632:string)  [unwired: 3 in]
                          n782 = Build Array(w1647, w1646, w1645, w1640, w1631, w1642, w1632) -> (w1643:string[])
                        }
                      }
                    }
                  }
                }
              }
              n783 = call "TestPlan - Config File.vi"("Action"=enum16{"Write", "Read", "Read All", "Remove"}."Write", "file path"=w1141, "error in (no error)"=w1140, "Value"=w1135, "Key Name"=w1138, "TestPlan Section"=w1139) -> ("error out"=w1142:errorcluster)  [unwired: 3 in, 2 out]
            }
            n784 = case shown="No Error" w1122 {
              selector: w1122 -> [w1129 w1132]
              tunnel: [w1129 w1132] -> w1121
              tunnel: [Test_Plan_Template_-_State."Close" ("Enum") Test_Plan_Template_-_State."Idle" ("Enum")] -> w1120
              frame No Error {
                n785 = One Button Dialog(message="Save Success") -> ()  [unwired: 1 in, 1 out]
              }
              frame Error {
              }
            }
          }
          frame "Close" {
          }
        }
      }
      frame Error {
        n786 = call <vilib>:"Clear Errors.vi"("error in (no error)"=w1656) -> ("error out"=w1655:errorcluster)  [unwired: 5 in, 1 out]
        n787 = Wait (ms)(milliseconds to wait=u32 100) -> ()  [unwired: 1 out]
      }
    }
  }
  "error out" <- w4
